vi "Display Module 2014.vi"(7 "Callling VI":refnum<vi>) -> ()   [LabVIEW 2016]
uses:
  Display Module TypeDefs/IMAQ Z Scale Bar.ctl
  <vilib>/Utility/miscctls.llb/LVPointTypeDef.ctl
  <vilib>/vision/Image Controls.llb/IMAQ Image.ctl
  <vilib>/Utility/miscctls.llb/LVRectTypeDef.ctl
  Display Module TypeDefs/Display Module Standard Action.ctl
  <vilib>/event_ctls.llb/lveventtype.ctl
  <vilib>/vision/NI_Vision_Development_Module.lvlib
panel:
  in  "Z Scale Channel 6":T1
  in  "Z Scale Channel 5":T1
  in  "Z Scale Channel 4":T1
  in  "Z Scale Channel 3":T1
  in  "Z Scale Channel 2":T1
  in  "Z Scale Channel 1":T1
  out "Messages":string
  in  "Max Left":bool
  in  "Max Right":bool
  in  "Add Display":bool
  in  "Remove Display":bool
  in  "Exit":bool
  out "Channel 6":T2(plugin-control)
  out "Channel 5":T2(plugin-control)
  out "Channel 4":T2(plugin-control)
  out "Channel 3":T2(plugin-control)
  out "Channel 2":T2(plugin-control)
  out "Channel 1":T2(plugin-control)
  # "Copyright (C) 2020 Edward S Allgeyer\n\nRedistribution and use in source and binary forms, with or without\nmodification, are permitted provided that the following conditions\nare met:\n\n1. Redistributions of source code must retain the above copyright\n   notice, this list of conditions and the following disclaimer.\n\n2. Redistributions in binary form must reproduce the above copyright\n   notice, this list of conditions and the following disclaimer in\n   the documentation and/or other materials provided with the\n   distribution.\n\n3. Neither the name of the copyright holder nor the names of its\n   contributors may be used to endorse or promote products derived\n   from this software without specific prior written permission.\n\nTHIS SOFTWARE IS PROVIDED BY THE COPYRIGHT HOLDERS AND CONTRIBUTORS\n\"AS IS\" AND ANY EXPRESS OR IMPLIED WARRANTIES, INCLUDING, BUT NOT\nLIMITED TO, THE IMPLIED WARRANTIES OF MERCHANTABILITY AND FITNESS\nFOR A PARTICULAR PURPOSE ARE DISCLAIMED. IN NO EVENT SHALL THE\nCOPYRIGHT HOLDER OR CONTRIBUTORS BE LIABLE FOR ANY DIRECT, INDIRECT,\nINCIDENTAL, SPECIAL, EXEMPLARY, OR CONSEQUENTIAL DAMAGES (INCLUDING,\nBUT NOT LIMITED TO, PROCUREMENT OF SUBSTITUTE GOODS OR SERVICES;\nLOSS OF USE, DATA, OR PROFITS; OR BUSINESS INTERRUPTION) HOWEVER\nCAUSED AND ON ANY THEORY OF LIABILITY, WHETHER IN CONTRACT, STRICT\nLIABILITY, OR TORT (INCLUDING NEGLIGENCE OR OTHERWISE) ARISING IN\nANY WAY OUT OF THE USE OF THIS SOFTWARE, EVEN IF ADVISED OF THE\nPOSSIBILITY OF SUCH DAMAGE."
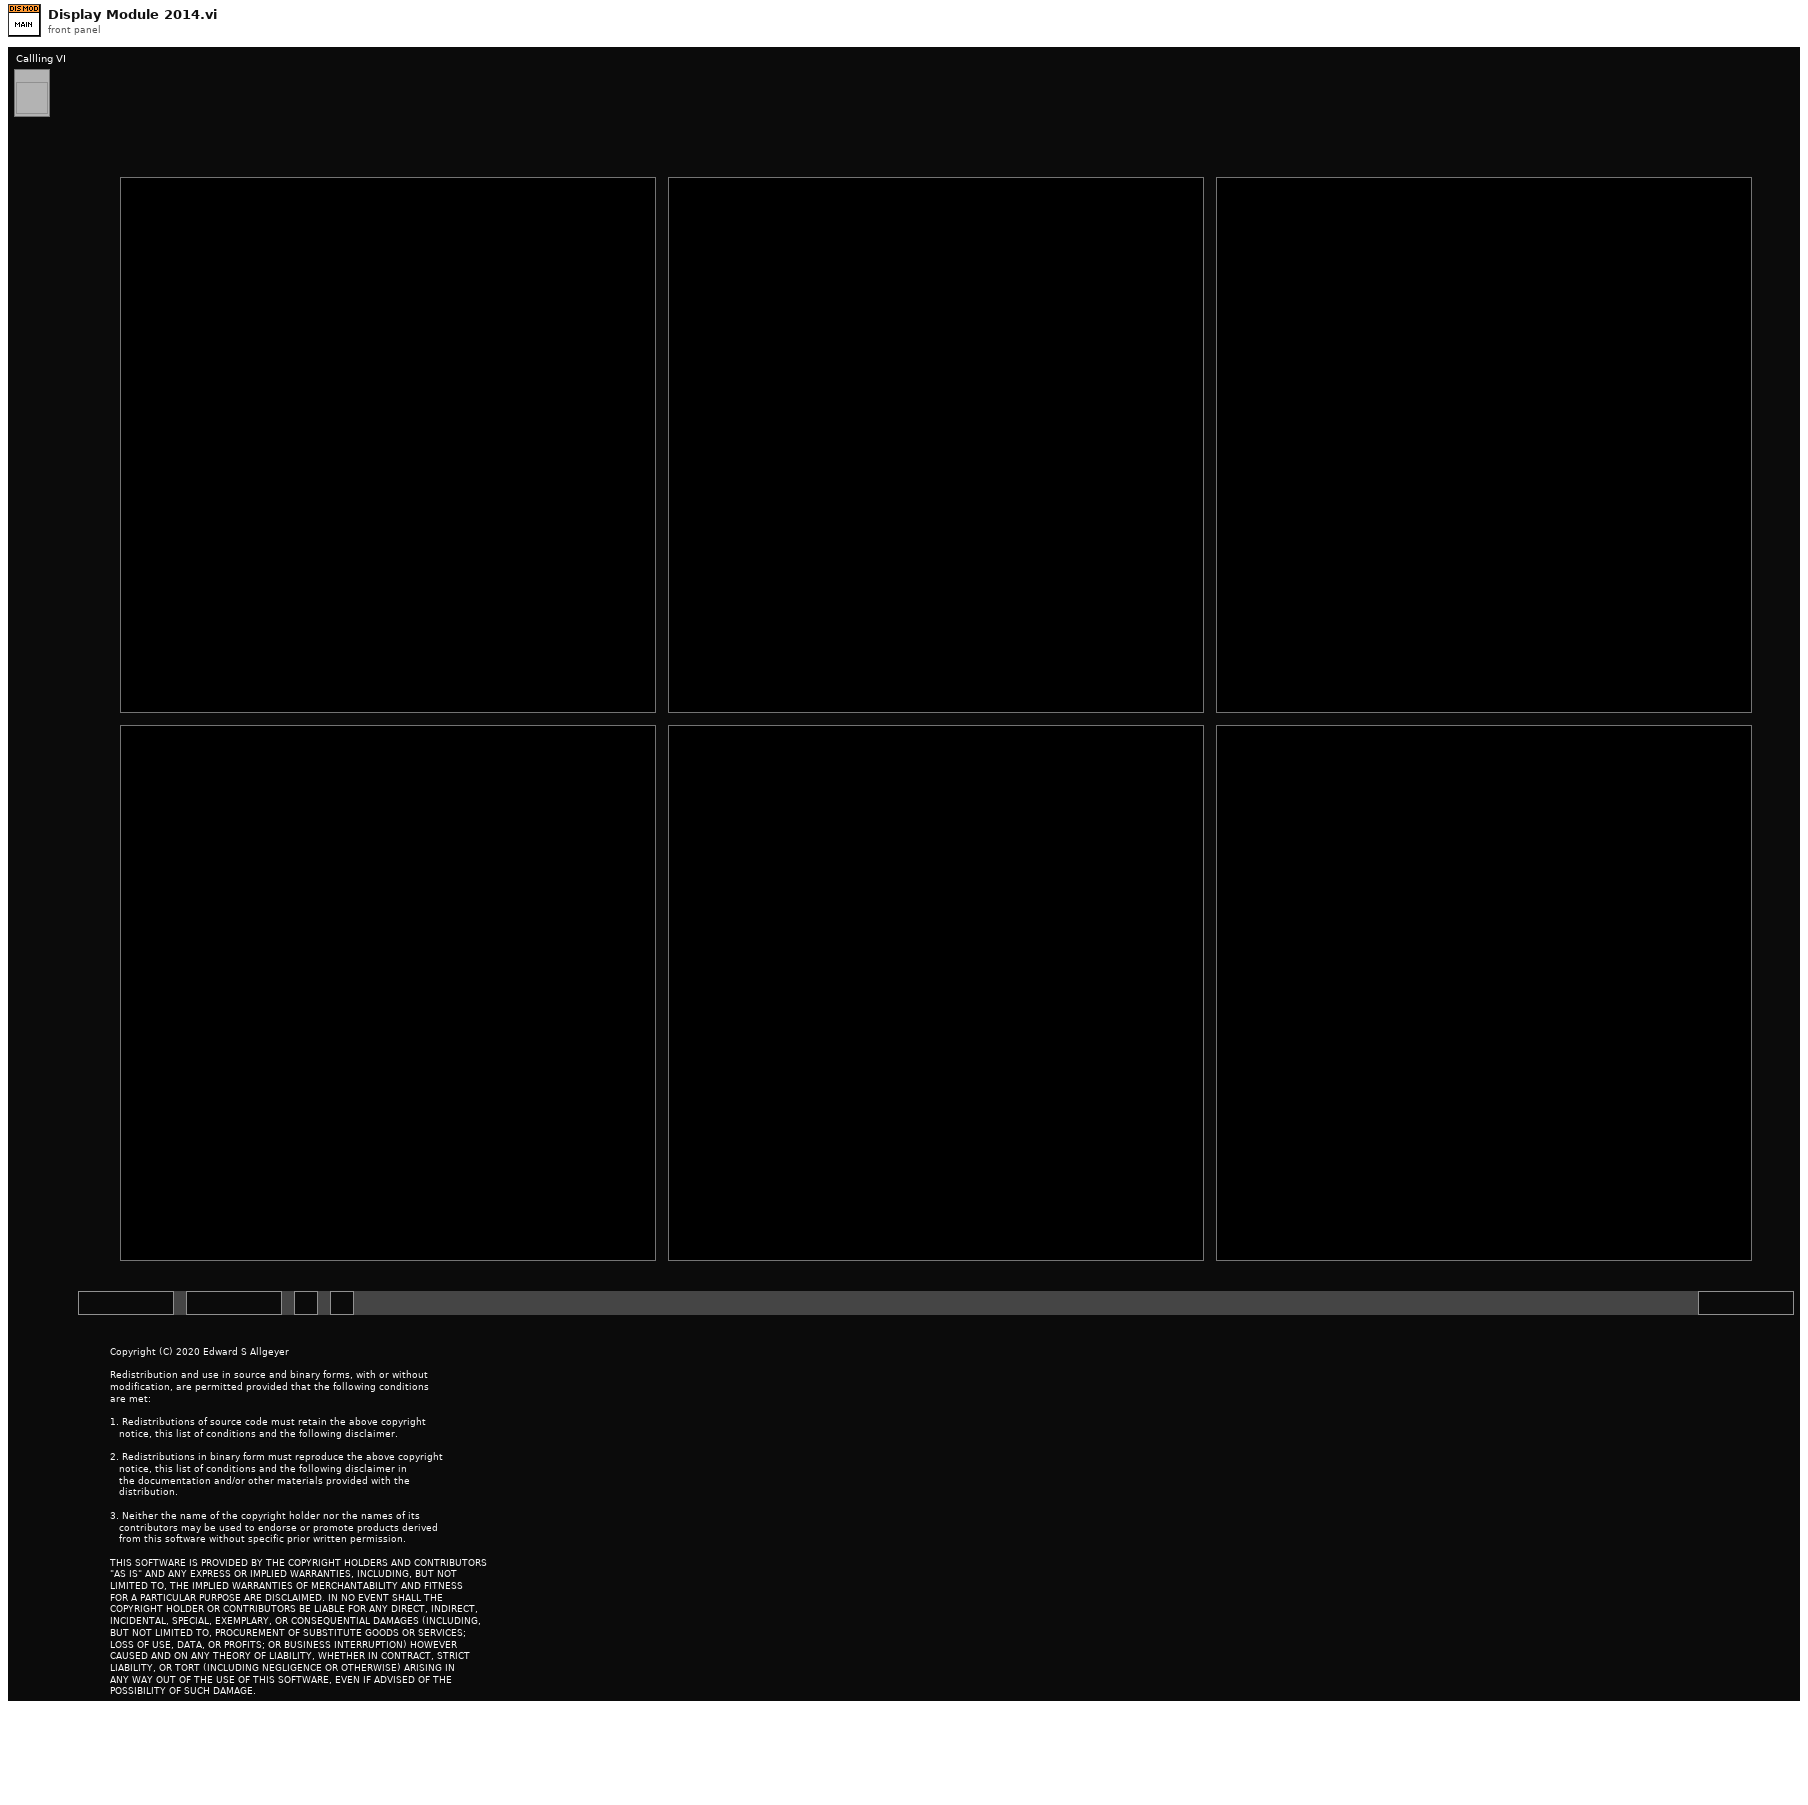
[diagram p1: front panel]
types:
  T1 = typedef "IMAQ Z Scale Bar.ctl" = cluster{"Z Scale Image":T2, "Z Scale Min":sgl, "Z Scale Max":sgl}
  T2 = typedef "IMAQ Image.ctl" = refnum<image>
  T3 = typedef "Image Type" = u32
  T4 = typedef "LVPointTypeDef.ctl" = cluster{"Horizontal":i16, "Vertical":i16}
  T5 = enum32{"Invalid", "Standard", "Closed", "Hidden", "Minimized", "Maximized"}
  T6 = enum16{"Always On", "Always Off", "Off While Running"}
  T7 = typedef "Display Module Standard Action.ctl" = enum16{"Read", "Write"}
  T8 = enum16{"Change Number", "Refresh Positions", "Get No. of Displays"}
  T9 = typedef "LVRectTypeDef.ctl" = cluster{"Left":i16, "Top":i16, "Right":i16, "Bottom":i16}
  T10 = typedef "lveventtype.ctl" = enum32{"Null", "Timeout", "Annotation Menu Selection", "Annotation Menu Selection?", "App Instance Close", "App Instance Close?", "Autoscale Range Change", "Bookmark Info Change", "Cell Edit", "Cell Edit?", "Cursor Grab", "Cursor Grab?", "Cursor Menu Selection", "Cursor Menu Selection?", "Cursor Move", "Cursor Release", "Data Change", "Direction Change", "Display State Change", "Drag Ended", "Drag Enter", "Drag Leave", "Drag Over", "Drag Source Update", "Drag Starting", "Drag Starting?", "Drop", "Exec State Change", "Key Down", "Key Down?", "Key Repeat", "Key Repeat?", "Key Up", "Listbox Double Click", "Menu Activation?", "Menu Selection (App)", "Menu Selection? (App)", "Menu Selection (User)", "Mouse Down", "Mouse Down?", "Mouse Enter", "Mouse Leave", "Mouse Move", "Mouse Up", "Mouse Wheel", "NI Security User Change (App)", "Pane Size", "Panel Close", "Panel Close?", "Panel Resize", "Plot Attribute Change", "Scale Range Change", "Shortcut Menu Activation?", "Shortcut Menu Selection (App)", "Shortcut Menu Selection? (App)", "Shortcut Menu Selection (User)", "Tree Double Click", "Tree Drag", "Tree Drag?", "Tree Drop", "Tree Drop?", "Tree Item Close", "Tree Item Close?", "Tree Item Open", "Tree Item Open?", "User Event", "Value Change"}
  T11 = cluster{"Global Rectangle":i32[], "Contours":cluster{"Contour Type":u32, "ROI Type":u32, "Points":i32[]}[]}
  T12 = typedef "LVAllMonitorsDisplayTypeDef.ctl" = cluster{"Bounds":cluster{"Left":i16, "Top":i16, "Right":i16, "Bottom":i16}, "Depth":i16}[]
  T13 = cluster{"Bounds":cluster{"Left":i16, "Top":i16, "Right":i16, "Bottom":i16}, "Depth":i16}
  T14 = cluster{"Mean Value":sgl, "Standard Variation":sgl, "Minimal Value":sgl, "Maximal Value":sgl, "Area (calibrated)":sgl, "Area (pixels)":u32, "%":sgl, "Calibration Valid":bool}
  T15 = cluster{"Contour Type":u32, "ROI Type":u32, "Points":i32[]}[]
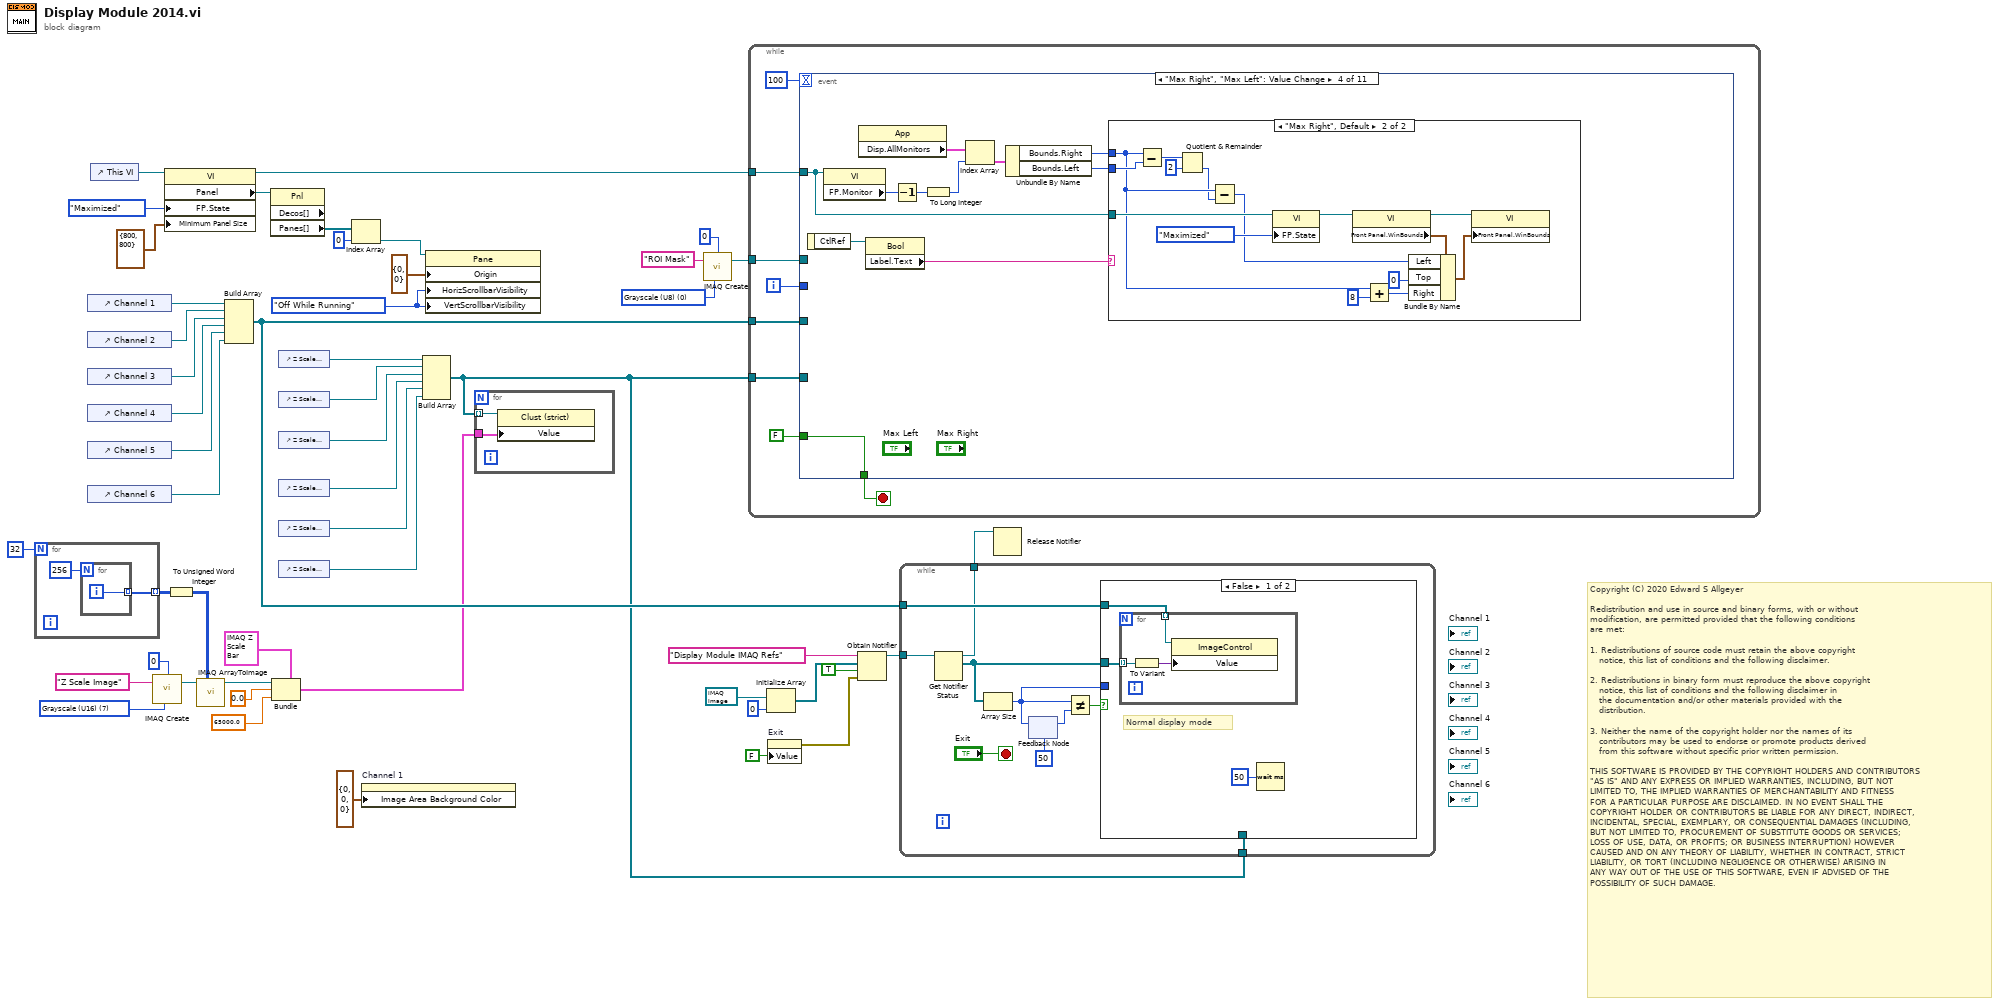
[diagram p0: block diagram]
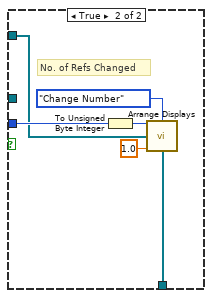
[diagram p2: hidden frame]
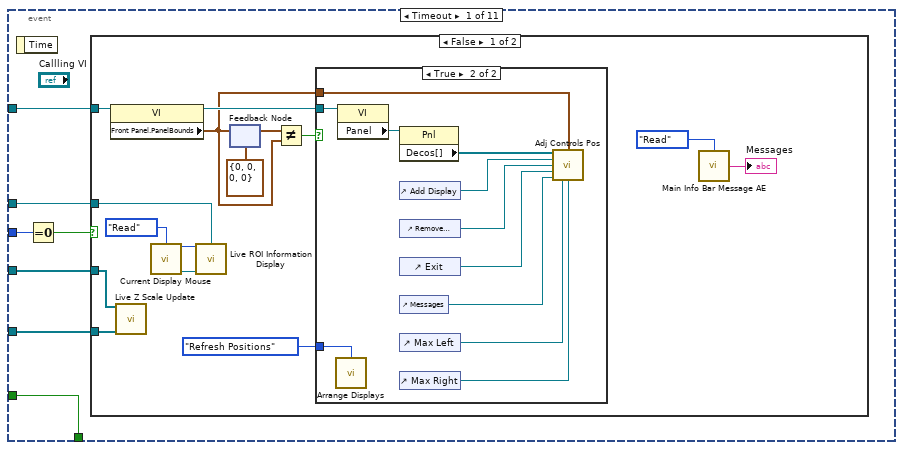
[diagram p3: hidden frame]
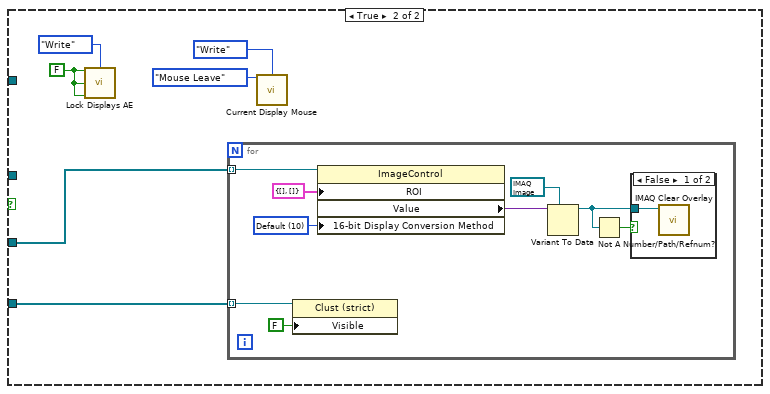
[diagram p5: hidden frame]
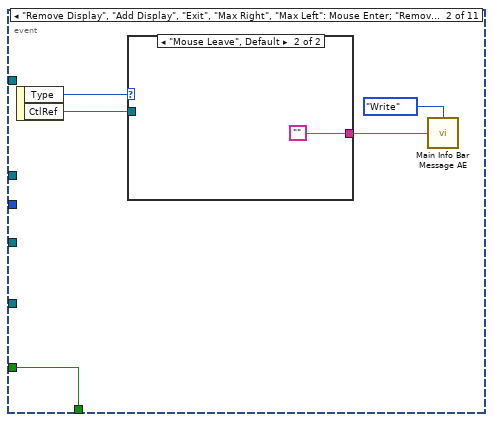
[diagram p7: hidden frame]
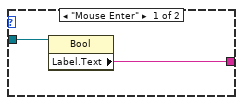
[diagram p8: hidden frame]
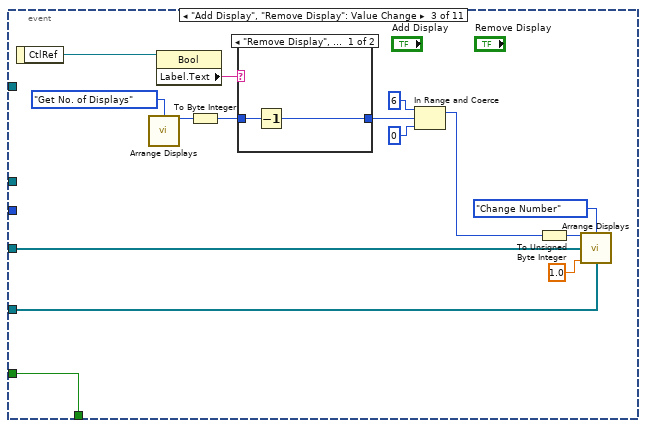
[diagram p9: hidden frame]
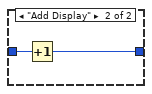
[diagram p10: hidden frame]
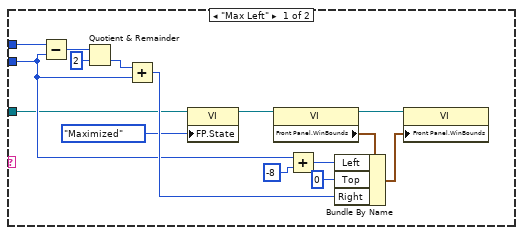
[diagram p11: hidden frame]
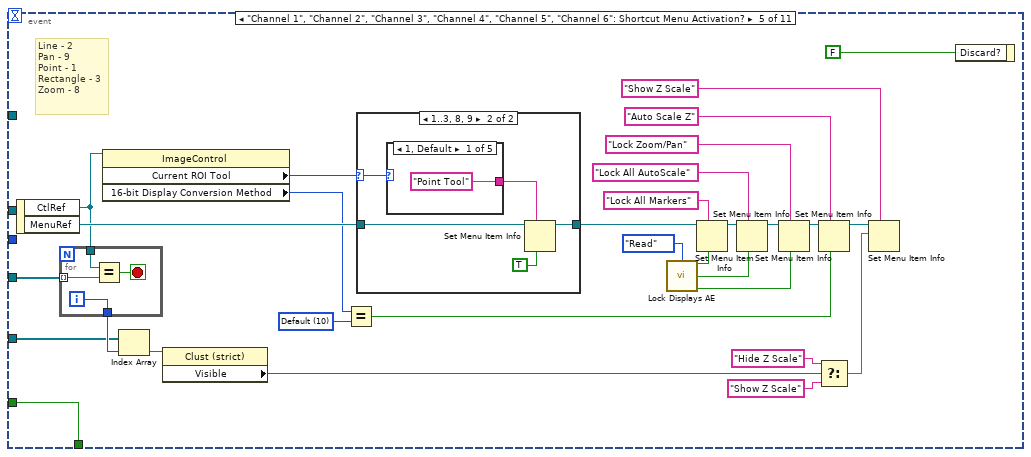
[diagram p12: hidden frame]
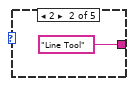
[diagram p14: hidden frame]
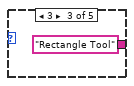
[diagram p15: hidden frame]
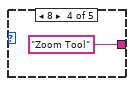
[diagram p16: hidden frame]
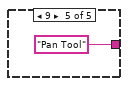
[diagram p17: hidden frame]
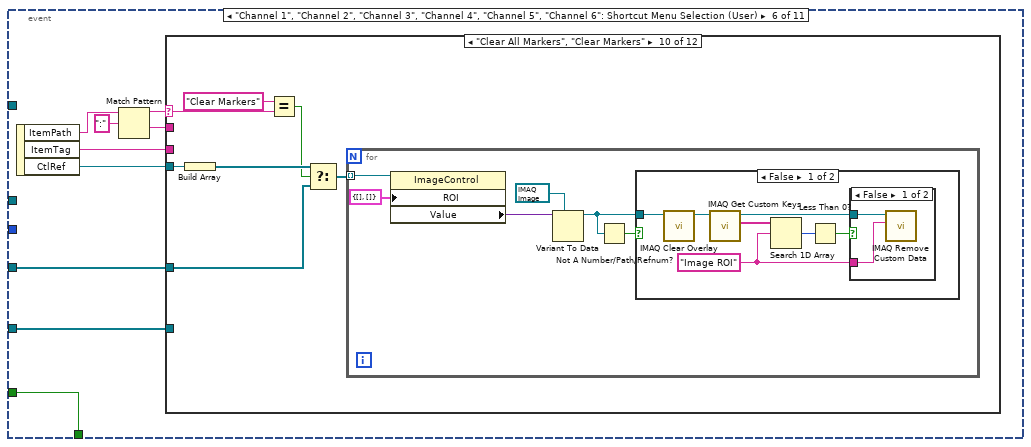
[diagram p18: hidden frame]
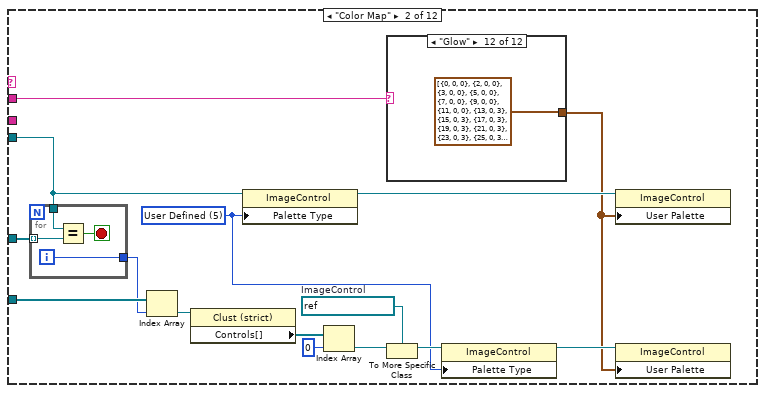
[diagram p20: hidden frame]
diagram:
  w20 = T3 7 items=["Grayscale (U8)", "Grayscale (I16)", "Grayscale (SGL)", "Complex (CSG)", "RGB (U32)", "HSL (U32)", "RGB (U64)", "Grayscale (U16)"] ("Image Type")
  w26 = T3 0 items=["Grayscale (U8)", "Grayscale (I16)", "Grayscale (SGL)", "Complex (CSG)", "RGB (U32)", "HSL (U32)", "RGB (U64)", "Grayscale (U16)"] ("Image Type")
  w41 = T6."Off While Running" ("Vertical Scrollbar Visibility")
  # "Copyright (C) 2020 Edward S Allgeyer\n\nRedistribution and use in source and binary forms, with or without\nmodification, are permitted provided that the following conditions\nare met:\n\n1. Redistributions of source code must retain the above copyright\n   notice, this list of conditions and the following disclaimer.\n\n2. Redistributions in binary form must reproduce the above copyright\n   notice, this list of conditions and the following disclaimer in\n   the documentation and/or other materials provided with the\n   distribution.\n\n3. Neither the name of the copyright holder nor the names of its\n   contributors may be used to endorse or promote products derived\n   from this software without specific prior written permission.\n\nTHIS SOFTWARE IS PROVIDED BY THE COPYRIGHT HOLDERS AND CONTRIBUTORS\n\"AS IS\" AND ANY EXPRESS OR IMPLIED WARRANTIES, INCLUDING, BUT NOT\nLIMITED TO, THE IMPLIED WARRANTIES OF MERCHANTABILITY AND FITNESS\nFOR A PARTICULAR PURPOSE ARE DISCLAIMED. IN NO EVENT SHALL THE\nCOPYRIGHT HOLDER OR CONTRIBUTORS BE LIABLE FOR ANY DIRECT, INDIRECT,\nINCIDENTAL, SPECIAL, EXEMPLARY, OR CONSEQUENTIAL DAMAGES (INCLUDING,\nBUT NOT LIMITED TO, PROCUREMENT OF SUBSTITUTE GOODS OR SERVICES;\nLOSS OF USE, DATA, OR PROFITS; OR BUSINESS INTERRUPTION) HOWEVER\nCAUSED AND ON ANY THEORY OF LIABILITY, WHETHER IN CONTRACT, STRICT\nLIABILITY, OR TORT (INCLUDING NEGLIGENCE OR OTHERWISE) ARISING IN\nANY WAY OUT OF THE USE OF THIS SOFTWARE, EVEN IF ADVISED OF THE\nPOSSIBILITY OF SUCH DAMAGE."
  n1 = for {
    N: 32 -> [_]
    tunnel: [w51] -> w18 mode=indexing
    n2 = for {
      N: 256 -> [_]
      tunnel: [w53] -> w51 mode=indexing
      i -> [w53]
    }
  }
  n3 = control-ref of="Channel 1"() -> (w50:refnum<vi>)
  n4 = control-ref of="Channel 2"() -> (w45:refnum<vi>)
  n5 = control-ref of="Channel 3"() -> (w46:refnum<vi>)
  n6 = control-ref of="Channel 4"() -> (w47:refnum<vi>)
  n7 = control-ref of="Channel 5"() -> (w48:refnum<vi>)
  n8 = control-ref of="Channel 6"() -> (w49:refnum<vi>)
  n9 = control-ref of="This VI"() -> (w40:refnum<vi>)
  n10 = call "IMAQ Create"("Border Size"=0, "Image Name"="Z Scale Image", "Image Type"=w20) -> ("New Image"=w19:T2)  [unwired: 2 in, 1 out]
  n11 = property class="VI"(reference=w40, "FP.State"=T5."Maximized" ("Front Panel Window:State"), "Minimum Panel Size"=T4 {"Horizontal"=800, "Vertical"=800} ("Front Panel Window:Minimum Size")) -> (reference out=w35:refnum<vi>, "Panel"=w36:refnum<vi>)  [unwired: 1 in, 1 out]
  n12 = To Unsigned Word Integer(number=w18) -> (unsigned 16bit integer=w17:u16[][])
  n13 = call "IMAQ ArrayToImage"("Image Pixels (U16)"=w17, "Image"=w19) -> ("Image Out"=w16:T2)  [unwired: 8 in, 1 out]
  n14 = Build Array(w50, w45, w46, w47, w48, w49) -> (w29:refnum<vi>[])
  n15 = property class="Pnl" props=["Decos[]", "Panes[]"](reference=w36) -> ("Panes[]"=w37:refnum<vi>[])  [unwired: 1 in, 3 out]
  n16 = Bundle(cluster=T1 {"Z Scale Image"="remote image 000000002503C6CC", "Z Scale Min"=0.0, "Z Scale Max"=65000.0} ("Z Scale Channel 6"), "Z Scale Image"=w16, "Z Scale Min"=sgl 0.0, "Z Scale Max"=sgl 65000.0) -> (w7:T1)
  n17 = control-ref of="Z Scale Channel 1"() -> (w13:refnum<vi>)
  n18 = control-ref of="Z Scale Channel 2"() -> (w8:refnum<vi>)
  n19 = control-ref of="Z Scale Channel 3"() -> (w9:refnum<vi>)
  n20 = control-ref of="Z Scale Channel 4"() -> (w10:refnum<vi>)
  n21 = control-ref of="Z Scale Channel 5"() -> (w11:refnum<vi>)
  n22 = control-ref of="Z Scale Channel 6"() -> (w12:refnum<vi>)
  n23 = Index Array(array=w37, index=0) -> (element=w43:refnum<vi>)
  n24 = property on="Channel 1" class="ImageControl"("Image Area Background Color"=cluster{"Red":u8, "Green":u8, "Blue":u8} {"Red"=0, "Green"=0, "Blue"=0} ("Image Area:Background:Background Color")) -> ()  [unwired: 2 in, 2 out]
  n25 = Build Array(w13, w8, w9, w10, w11, w12) -> (w5:refnum<vi>[])
  n26 = property class="Pane"(reference=w43, "Origin"=T4 {"Horizontal"=0, "Vertical"=0}, "HorizScrollbarVisibility"=w41, "VertScrollbarVisibility"=w41) -> ()  [unwired: 1 in, 2 out]
  n27 = for {
    tunnel: w5 -> [w55] mode=indexing
    tunnel: w7 -> [w54]
    n28 = property class="Clust (strict)"(reference=w55, "Value"=w54) -> ()  [unwired: 1 in, 2 out]
  }
  n29 = call "IMAQ Create"("Border Size"=0, "Image Name"="ROI Mask", "Image Type"=w26) -> ("New Image"=w24:T2)  [unwired: 2 in, 1 out]
  n30 = while {
    tunnel: w29 -> [w62]
    tunnel: w35 -> [w58]
    tunnel: w24 -> [w57]
    tunnel: w5 -> [w56]
    i -> [w63]
    stop <- w61 stop-if-true
    n31 = event shown="[3] \"Max Right\", \"Max Left\": Value Change" {
      selector: _ -> [_ _ _ _ _ _ _ _ _ _ _]
      dyn-events: _ -> [_ _ _ _ _ _ _ _ _ _ _]
      timeout: 100 -> [_ _ _ _ _ _ _ _ _ _ _]
      tunnel: w63 -> [w70 _ _ _ _ _ _ _ _ _ _]
      tunnel: w62 -> [w68 _ w122 _ w185 w228 w397 _ w433 w441 w458]
      tunnel: [w67 w117 w135 w150 w209 w234 w402 w424 w435 w447 w459] -> w61
      tunnel: FALSE -> [w67 w117 w135 w150 w209 w234 w402 w424 w435 w447 _]
      tunnel: w58 -> [w66 _ _ w141 _ _ _ _ _ _ _]
      tunnel: w57 -> [w65 _ _ _ _ _ _ _ _ _ w457]
      tunnel: w56 -> [w64 _ w123 _ w186 w227 _ _ w434 _ _]
      event Timeout {
        n32 = event-data() -> ()  [unwired: 1 in, 1 out]
        n33 = Equal To 0?(x=w70) -> (x = 0?=w69:bool)
        n34 = case shown="False" w69 {
          tunnel: w68 -> [w72 w100]
          tunnel: w66 -> [w85 _]
          tunnel: w65 -> [w78 _]
          tunnel: w64 -> [w71 w99]
          frame False {
            n35 = property class="VI"(reference=w85) -> (reference out=w81:refnum<vi>, "Front Panel.PanelBounds"=w80:T9)  [unwired: 1 in, 1 out]
            n36 = call "Live Z Scale Update.vi"("IMAQ Display Refs"=w72, "Z Scale Refs"=w71) -> ()  [unwired: 14 in]
            n37 = call "Current Display Mouse.vi"("Action"=Display_Module_Standard_Action."Read") -> ("Event Type Out"=w76:T10, "IMAQ Image Display Ref Out"=w75:refnum<vi>)  [unwired: 13 in]
            n38 = call "Live ROI Information Display.vi"("Event Type"=w76, "ROI Mask REF"=w78, "IMAQ Image Display Ref"=w75) -> ()  [unwired: 13 in]
            n39 = feedback-in #1(w80) -> ()
            n40 = feedback #1(T9 {"Left"=0, "Top"=0, "Right"=0, "Bottom"=0} ("Front Panel.PanelBounds")) -> (w84:T9)
            n41 = Not Equal?(x=w84, y=w80) -> (x != y?=w82:bool)
            n42 = case shown="True" w82 {
              tunnel: w81 -> [_ w90]
              tunnel: w80 -> [_ w89]
              tunnel: T8."Refresh Positions" ("Action") -> [_ w86]
              frame False {
              }
              frame True {
                n43 = call "Arrange Displays.vi"("Action"=w86) -> ()  [unwired: 13 in, 2 out]
                n44 = property class="VI"(reference=w90) -> ("Panel"=w96:refnum<vi>)  [unwired: 1 in, 2 out]
                n45 = property class="Pnl"(reference=w96) -> ("Decos[]"=w95:refnum<vi>[])  [unwired: 1 in, 2 out]
                n46 = control-ref of="Add Display"() -> (w91:refnum<vi>)
                n47 = control-ref of="Remove Display"() -> (w94:refnum<vi>)
                n48 = control-ref of="Exit"() -> (w93:refnum<vi>)
                n49 = control-ref of="Messages"() -> (w92:refnum<vi>)
                n50 = control-ref of="Max Left"() -> (w88:refnum<vi>)
                n51 = control-ref of="Max Right"() -> (w87:refnum<vi>)
                n52 = call "Adj Controls Pos.vi"("Decoration Ref Array"=w95, "Panel Bounds"=w89, "Add Display Ref (Bool)"=w91, "Remove Display Ref (Bool)"=w94, "Exit (Bool)"=w93, "Message (String)"=w92, "Max Left (Bool)"=w88, "Max Right (Bool)"=w87) -> ()  [unwired: 8 in]
              }
            }
            n53 = call "Main Info Bar Message AE.vi"("Action"=Display_Module_Standard_Action."Read") -> ("Message Out"=→"Messages":string)  [unwired: 14 in]
          }
          frame True {
            w102 = FALSE ("Lock All Markers")
            n54 = call "Lock Displays AE.vi"("Lock All Markers"=w102, "Action"=Display_Module_Standard_Action."Write", "Lock All AutoScale"=w102, "Lock Pan/Zoom"=w102) -> ()  [unwired: 9 in, 3 out]
            n55 = for {
              tunnel: w100 -> [w106] mode=indexing
              tunnel: w99 -> [w105] mode=indexing
              w103 = u32 10 items=["Default"=10, "Most Significant Bits"=11, "Full Dynamic"=12, "Downshift"=13, "Given Range"=14, "90% Dynamic"=15, "Given Percent Range"=16] ("16-bit Display Mapping:Conversion Method")
              n56 = property class="Clust (strict)"(reference=w105, "Visible"=FALSE) -> ()  [unwired: 1 in, 2 out]
              n57 = property class="ImageControl"(reference=w106, "ROI"=T11 {"Global Rectangle"=[], "Contours"=[]}, "16-bit Display Conversion Method"=w103) -> ("Value"=w107:variant)  [unwired: 1 in, 2 out]
              n58 = Variant To Data(type=T2 refnum ("New Image"), Variant=w107) -> (data=w110:T2)  [unwired: 1 in, 1 out]
              n59 = Not A Number/Path/Refnum?(number/path/refnum=w110) -> (NaN/Path/Refnum?=w109:bool)
              n60 = case shown="False" w109 {
                tunnel: w110 -> [w112 _]
                frame False {
                  n61 = call "IMAQ Clear Overlay"("Image"=w112) -> ()  [unwired: 9 in, 2 out]
                }
                frame True {
                }
              }
            }
            n62 = call "Current Display Mouse.vi"("Event Type"=lveventtype."Mouse Leave", "Action"=Display_Module_Standard_Action."Write") -> ()  [unwired: 12 in, 2 out]
          }
        }
      }
      event "Remove Display", "Add Display", "Exit", "Max Right", "Max Left": Mouse Enter; "Remove Display", "Add Display", "Exit", "Max Right", "Max Left": Mouse Leave {
        n63 = event-data() -> ("Type"=w116:T10, "CtlRef"=w115:refnum<vi>)  [unwired: 1 in]
        n64 = case shown="\"Mouse Leave\", Default" w116 {
          tunnel: w115 -> [w119 _]
          tunnel: [w118 ""] -> w113
          frame "Mouse Enter" {
            n65 = property class="Bool"(reference=w119) -> ("Label.Text"=w118:string)  [unwired: 1 in, 2 out]
          }
          frame "Mouse Leave", Default {
          }
        }
        n66 = call "Main Info Bar Message AE.vi"("Action"=Display_Module_Standard_Action."Write", "Message"=w113) -> ()  [unwired: 13 in, 1 out]
      }
      event "Add Display", "Remove Display": Value Change {
        n67 = event-data() -> ("CtlRef"=w134:refnum<vi>)  [unwired: 1 in]
        n68 = call "Arrange Displays.vi"("Action"=T8."Get No. of Displays") -> ("Number of Displays Out"=w125:u8)  [unwired: 13 in, 1 out]
        n69 = property class="Bool"(reference=w134) -> ("Label.Text"=w133:string)  [unwired: 1 in, 2 out]
        n70 = To Byte Integer(number=w125) -> (8bit integer=w124:i8)
        n71 = case shown="\"Remove Display\", Default" w133 {
          tunnel: w124 -> [w137 w139]
          tunnel: [w136 w138] -> w130
          frame "Remove Display", Default {
            n72 = Decrement(x=w137) -> (x-1=w136:i8)
          }
          frame "Add Display" {
            n73 = Increment(x=w139) -> (x+1=w138:i8)
          }
        }
        n74 = In Range and Coerce(upper limit=i8 6, x=w130, lower limit=i8 0) -> (coerced(x)=w129:i8)  [unwired: 1 out]
        n75 = To Unsigned Byte Integer(number=w129) -> (unsigned 8bit integer=w128:u8)
        n76 = call "Arrange Displays.vi"("Number of Displays"=w128, "Action"=T8."Change Number", "IMAQ Display Refs"=w122, "Aspect Ratio (Width/Height)"=1.0, "Z Scale Refs"=w123) -> ()  [unwired: 9 in, 2 out]
      }
      event "Max Right", "Max Left": Value Change {
        n77 = event-data() -> ("CtlRef"=w149:refnum<vi>)  [unwired: 1 in]
        n78 = property class="VI"(reference=w141) -> ("FP.Monitor"=w148:u16)  [unwired: 1 in, 2 out]
        n79 = property class="App"() -> ("Disp.AllMonitors"=w147:T12)  [unwired: 2 in, 2 out]
        n80 = property class="Bool"(reference=w149) -> ("Label.Text"=w140:string)  [unwired: 1 in, 2 out]
        n81 = Decrement(x=w148) -> (x-1=w146:u16)
        n82 = To Long Integer(number=w146) -> (32bit integer=w145:i32)
        n83 = Index Array(array=w147, index=w145) -> (element=w144:T13)
        n84 = Unbundle By Name(w144) -> ("Bounds.Right"=w143:i16, "Bounds.Left"=w142:i16)
        n85 = case shown="\"Max Right\", Default" w140 {
          tunnel: w143 -> [w165 w168]
          tunnel: w142 -> [w153 w172]
          tunnel: w141 -> [w151 w171]
          frame "Max Left" {
            n86 = Subtract(x=w165, y=w153) -> (x-y=w160:i16)
            n87 = Quotient & Remainder(x=w160, y=i16 2) -> (floor(x/y)=w158:i16)  [unwired: 1 out]
            n88 = Add(x=w158, y=w153) -> (x+y=w157:i16)
            n89 = property class="VI"(reference=w151, "FP.State"=T5."Maximized" ("Front Panel Window:State")) -> (reference out=w155:refnum<vi>)  [unwired: 1 in, 1 out]
            n90 = property class="VI"(reference=w155) -> (reference out=w164:refnum<vi>, "Front Panel.WinBounds"=w162:T9)  [unwired: 1 in, 1 out]
            n91 = Add(x=w153, y=i16 -8 ("Left")) -> (x+y=w152:i16)
            n92 = Bundle By Name(cluster=w162, "Left"=w152, "Top"=i16 0, "Right"=w157) -> (w163:T9)
            n93 = property class="VI"(reference=w164, "Front Panel.WinBounds"=w163) -> ()  [unwired: 1 in, 2 out]
          }
          frame "Max Right", Default {
            n94 = Subtract(x=w168, y=w172) -> (x-y=w177:i16)
            n95 = Quotient & Remainder(x=w177, y=i16 2) -> (floor(x/y)=w167:i16)  [unwired: 1 out]
            n96 = Subtract(x=w168, y=w167) -> (x-y=w166:i16)
            n97 = property class="VI"(reference=w171, "FP.State"=T5."Maximized" ("Front Panel Window:State")) -> (reference out=w174:refnum<vi>)  [unwired: 1 in, 1 out]
            n98 = property class="VI"(reference=w174) -> (reference out=w180:refnum<vi>, "Front Panel.WinBounds"=w178:T9)  [unwired: 1 in, 1 out]
            n99 = Add(x=w168, y=i16 8 ("Left")) -> (x+y=w169:i16)
            n100 = Bundle By Name(cluster=w178, "Left"=w166, "Top"=i16 0, "Right"=w169) -> (w179:T9)
            n101 = property class="VI"(reference=w180, "Front Panel.WinBounds"=w179) -> ()  [unwired: 1 in, 2 out]
          }
        }
      }
      event "Channel 1", "Channel 2", "Channel 3", "Channel 4", "Channel 5", "Channel 6": Shortcut Menu Activation? {
        w192 = u32 10 items=["Default"=10, "Most Significant Bits"=11, "Full Dynamic"=12, "Downshift"=13, "Given Range"=14, "90% Dynamic"=15, "Given Percent Range"=16] ("16-bit Display Mapping:Conversion Method")
        # "Line - 2\nPan - 9\nPoint - 1\nRectangle - 3\nZoom - 8"
        n102 = event-data() -> ("CtlRef"=w187:refnum<vi>, "MenuRef"=w207:refnum<k9>)  [unwired: 1 in]
        n103 = for {
          tunnel: w185 -> [w214] mode=indexing
          tunnel: w187 -> [w212]
          tunnel: [w211] -> w189
          i -> [w211]
          stop <- w213 stop-if-true
          n104 = Equal?(x=w212, y=w214) -> (x = y?=w213:bool)
        }
        n105 = property class="ImageControl"(reference=w187) -> ("Current ROI Tool"=w208:u32, "16-bit Display Conversion Method"=w194:u32)  [unwired: 1 in, 2 out]
        n106 = Index Array(array=w186, index=w189) -> (element=w188:refnum<vi>)
        n107 = property class="Clust (strict)"(reference=w188) -> ("Visible"=w181:bool)  [unwired: 1 in, 2 out]
        n108 = Equal?(x=w194, y=w192) -> (x = y?=w193:bool)
        n109 = case shown="1..3, 8, 9" w208 {
          selector: w208 -> [_ w220]
          tunnel: w207 -> [w215 w218]
          tunnel: [w215 w216] -> w206
          frame Default {
          }
          frame 1..3, 8, 9 {
            n110 = case shown="1, Default" w220 {
              tunnel: ["Point Tool" ("item tag") "Line Tool" ("item tag") "Rectangle Tool" ("item tag") "Zoom Tool" ("item tag") "Pan Tool" ("item tag")] -> w217
              frame 1, Default {
              }
              frame 2 {
              }
              frame 3 {
              }
              frame 8 {
              }
              frame 9 {
              }
            }
            n111 = Set Menu Item Info(6:TRUE ("checked"), 7:w217, 11:w218) -> (3:w216:refnum<k9>)  [unwired: 4 in, 1 out]
          }
        }
        n112 = call "Lock Displays AE.vi"("Action"=Display_Module_Standard_Action."Read") -> ("Lock All Markers Out"=w199:bool, "Lock All AutoScale Out"=w198:bool, "Lock Pan/Zoom Out"=w197:bool)  [unwired: 12 in]
        n113 = Set Menu Item Info(6:w199, 7:"Lock All Markers" ("item tag"), 11:w206) -> (3:w205:refnum<k9>)  [unwired: 4 in, 1 out]
        n114 = Set Menu Item Info(6:w198, 7:"Lock All AutoScale" ("item tag"), 11:w205) -> (3:w204:refnum<k9>)  [unwired: 4 in, 1 out]
        n115 = Set Menu Item Info(6:w197, 7:"Lock Zoom/Pan" ("item tag"), 11:w204) -> (3:w196:refnum<k9>)  [unwired: 4 in, 1 out]
        n116 = Set Menu Item Info(6:w193, 7:"Auto Scale Z" ("item tag"), 11:w196) -> (3:w191:refnum<k9>)  [unwired: 4 in, 1 out]
        n117 = Select(t="Hide Z Scale" ("item tag"), s=w181, f="Show Z Scale" ("item tag")) -> (s? t:f=w182:string)
        n118 = Set Menu Item Info(7:"Show Z Scale" ("item tag"), 10:w182, 11:w191) -> ()  [unwired: 4 in, 2 out]
        n119 = event-data("Discard?"=FALSE) -> ()  [unwired: 1 in, 1 out]
      }
      event "Channel 1", "Channel 2", "Channel 3", "Channel 4", "Channel 5", "Channel 6": Shortcut Menu Selection (User) {
        n120 = event-data() -> ("ItemPath"=w232:string, "ItemTag"=w233:string, "CtlRef"=w229:refnum<vi>)  [unwired: 1 in]
        n121 = Match Pattern(string=w232, regular expression=":") -> (before substring=w230:string, after substring=w226:string)  [unwired: 1 in, 2 out]
        n122 = case shown="\"Clear All Markers\", \"Clear Markers\"" w230 {
          selector: w230 -> [_ _ w267 _ _ _ _ _ _ w363 _ _]
          tunnel: w229 -> [_ w247 w273 w298 _ w320 _ w334 w344 w361 w385 _]
          tunnel: w233 -> [_ _ _ _ _ _ _ _ _ _ _ _]
          tunnel: w228 -> [_ w248 _ w301 w312 w322 _ w333 w345 w359 w381 _]
          tunnel: w227 -> [_ w246 _ w300 _ w321 _ _ _ _ _ _]
          tunnel: w226 -> [_ w235 _ _ _ _ _ _ _ _ _ _]
          frame Default {
          }
          frame "Color Map" {
            w241 = refnum<vi> refnum  # ImageControl
            w237 = u32 5 items=["Grayscale", "Binary", "Gradient", "Rainbow", "Temperature", "User Defined", "Binary 16 Bit", "Gradient 16 Bit", "Rainbow 16 Bit", "Temperature 16 Bit", "User Defined 16 Bit"] ("Palette:Palette Type")
            n123 = for {
              tunnel: w248 -> [w264] mode=indexing
              tunnel: [w265] -> w245
              tunnel: w247 -> [w263]
              i -> [w265]
              stop <- w262 stop-if-true
              n124 = Equal?(x=w263, y=w264) -> (x = y?=w262:bool)
            }
            n125 = Index Array(array=w246, index=w245) -> (element=w244:refnum<vi>)
            n126 = property class="Clust (strict)"(reference=w244) -> ("Controls[]"=w243:refnum<vi>[])  [unwired: 1 in, 2 out]
            n127 = property class="ImageControl"(reference=w247, "Palette Type"=w237) -> (reference out=w249:refnum<vi>)  [unwired: 1 in, 1 out]
            n128 = Index Array(array=w243, index=0) -> (element=w240:refnum<vi>)
            n129 = case shown="\"Glow\"" w235 {
              tunnel: [cluster{u8, u8, u8}[] [{0, 0, 0}, {1, 1, 1}, {2, 2, 2}, {3, 3, 3}, {4, 4, 4}, {5, 5, 5}, {6, 6, 6}, {7, 7, 7}, {8, 8, 8}, {9, 9, 9}, {10, 10, 10}, {11, 11, 11}, {12, 12, 12}, {13, 13, 13}, {14, 14, 14}, {15, 15, 15}, {16, 16, 16}, {17, 17, 17}, {18, 18, 18}, {19, 19, 19}, {20, 20, 20}, {21, 21, 21}, {22, 22, 22}, {23, 23, 23}, {24, 24, 24}, {25, 25, 25}, {26, 26, 26}, {27, 27, 27}, {28, 28, 28}, {29, 29, 29}, {30, 30, 30}, {31, 31, 31}, {32, 32, 32}, {33, 33, 33}, {34, 34, 34}, {35, 35, 35}, {36, 36, 36}, {37, 37, 37}, {38, 38, 38}, {39, 39, 39}, {40, 40, 40}, {41, 41, 41}, {42, 42, 42}, {43, 43, 43}, {44, 44, 44}, {45, 45, 45}, {46, 46, 46}, {47, 47, 47}, {48, 48, 48}, {49, 49, 49}, {50, 50, 50}, {51, 51, 51}, {52, 52, 52}, {53, 53, 53}, {54, 54, 54}, {55, 55, 55}, {56, 56, 56}, {57, 57, 57}, {58, 58, 58}, {59, 59, 59}, {60, 60, 60}, {61, 61, 61}, {62, 62, 62}, {63, 63, 63}, {64, 64, 64}, {65, 65, 65}, {66, 66, 66}, {67, 67, 67}, {68, 68, 68}, {69, 69, 69}, {70, 70, 70}, {71, 71, 71}, {72, 72, 72}, {73, 73, 73}, {74, 74, 74}, {75, 75, 75}, {76, 76, 76}, {77, 77, 77}, {78, 78, 78}, {79, 79, 79}, {80, 80, 80}, {81, 81, 81}, {82, 82, 82}, {83, 83, 83}, {84, 84, 84}, {85, 85, 85}, {86, 86, 86}, {87, 87, 87}, {88, 88, 88}, {89, 89, 89}, {90, 90, 90}, {91, 91, 91}, {92, 92, 92}, {93, 93, 93}, {94, 94, 94}, {95, 95, 95}, {96, 96, 96}, {97, 97, 97}, {98, 98, 98}, {99, 99, 99}, {100, 100, 100}, {101, 101, 101}, {102, 102, 102}, {103, 103, 103}, {104, 104, 104}, {105, 105, 105}, {106, 106, 106}, {107, 107, 107}, {108, 108, 108}, {109, 109, 109}, {110, 110, 110}, {111, 111, 111}, {112, 112, 112}, {113, 113, 113}, {114, 114, 114}, {115, 115, 115}, {116, 116, 116}, {117, 117, 117}, {118, 118, 118}, {119, 119, 119}, {120, 120, 120}, {121, 121, 121}, {122, 122, 122}, {123, 123, 123}, {124, 124, 124}, {125, 125, 125}, {126, 126, 126}, {127, 127, 127}, {128, 128, 128}, {129, 129, 129}, {130, 130, 130}, {131, 131, 131}, {132, 132, 132}, {133, 133, 133}, {134, 134, 134}, {135, 135, 135}, {136, 136, 136}, {137, 137, 137}, {138, 138, 138}, {139, 139, 139}, {140, 140, 140}, {141, 141, 141}, {142, 142, 142}, {143, 143, 143}, {144, 144, 144}, {145, 145, 145}, {146, 146, 146}, {147, 147, 147}, {148, 148, 148}, {149, 149, 149}, {150, 150, 150}, {151, 151, 151}, {152, 152, 152}, {153, 153, 153}, {154, 154, 154}, {155, 155, 155}, {156, 156, 156}, {157, 157, 157}, {158, 158, 158}, {159, 159, 159}, {160, 160, 160}, {161, 161, 161}, {162, 162, 162}, {163, 163, 163}, {164, 164, 164}, {165, 165, 165}, {166, 166, 166}, {167, 167, 167}, {168, 168, 168}, {169, 169, 169}, {170, 170, 170}, {171, 171, 171}, {172, 172, 172}, {173, 173, 173}, {174, 174, 174}, {175, 175, 175}, {176, 176, 176}, {177, 177, 177}, {178, 178, 178}, {179, 179, 179}, {180, 180, 180}, {181, 181, 181}, {182, 182, 182}, {183, 183, 183}, {184, 184, 184}, {185, 185, 185}, {186, 186, 186}, {187, 187, 187}, {188, 188, 188}, {189, 189, 189}, {190, 190, 190}, {191, 191, 191}, {192, 192, 192}, {193, 193, 193}, {194, 194, 194}, {195, 195, 195}, {196, 196, 196}, {197, 197, 197}, {198, 198, 198}, {199, 199, 199}, {200, 200, 200}, {201, 201, 201}, {202, 202, 202}, {203, 203, 203}, {204, 204, 204}, {205, 205, 205}, {206, 206, 206}, {207, 207, 207}, {208, 208, 208}, {209, 209, 209}, {210, 210, 210}, {211, 211, 211}, {212, 212, 212}, {213, 213, 213}, {214, 214, 214}, {215, 215, 215}, {216, 216, 216}, {217, 217, 217}, {218, 218, 218}, {219, 219, 219}, {220, 220, 220}, {221, 221, 221}, {222, 222, 222}, {223, 223, 223}, {224, 224, 224}, {225, 225, 225}, {226, 226, 226}, {227, 227, 227}, {228, 228, 228}, {229, 229, 229}, {230, 230, 230}, {231, 231, 231}, {232, 232, 232}, {233, 233, 233}, {234, 234, 234}, {235, 235, 235}, {236, 236, 236}, {237, 237, 237}, {238, 238, 238}, {239, 239, 239}, {240, 240, 240}, {241, 241, 241}, {242, 242, 242}, {243, 243, 243}, {244, 244, 244}, {245, 245, 245}, {246, 246, 246}, {247, 247, 247}, {248, 248, 248}, {249, 249, 249}, {250, 250, 250}, {251, 251, 251}, {252, 252, 252}, {253, 253, 253}, {254, 254, 254}, {255, 255, 255}] ("Array") cluster{u8, u8, u8}[] [{0, 0, 0}, {1, 0, 0}, {2, 0, 0}, {3, 0, 0}, {4, 0, 0}, {5, 0, 0}, {6, 0, 0}, {7, 0, 0}, {8, 0, 0}, {9, 0, 0}, {10, 0, 0}, {11, 0, 0}, {12, 0, 0}, {13, 0, 0}, {14, 0, 0}, {15, 0, 0}, {16, 0, 0}, {17, 0, 0}, {18, 0, 0}, {19, 0, 0}, {20, 0, 0}, {21, 0, 0}, {22, 0, 0}, {23, 0, 0}, {24, 0, 0}, {25, 0, 0}, {26, 0, 0}, {27, 0, 0}, {28, 0, 0}, {29, 0, 0}, {30, 0, 0}, {31, 0, 0}, {32, 0, 0}, {33, 0, 0}, {34, 0, 0}, {35, 0, 0}, {36, 0, 0}, {37, 0, 0}, {38, 0, 0}, {39, 0, 0}, {40, 0, 0}, {41, 0, 0}, {42, 0, 0}, {43, 0, 0}, {44, 0, 0}, {45, 0, 0}, {46, 0, 0}, {47, 0, 0}, {48, 0, 0}, {49, 0, 0}, {50, 0, 0}, {51, 0, 0}, {52, 0, 0}, {53, 0, 0}, {54, 0, 0}, {55, 0, 0}, {56, 0, 0}, {57, 0, 0}, {58, 0, 0}, {59, 0, 0}, {60, 0, 0}, {61, 0, 0}, {62, 0, 0}, {63, 0, 0}, {64, 0, 0}, {65, 0, 0}, {66, 0, 0}, {67, 0, 0}, {68, 0, 0}, {69, 0, 0}, {70, 0, 0}, {71, 0, 0}, {72, 0, 0}, {73, 0, 0}, {74, 0, 0}, {75, 0, 0}, {76, 0, 0}, {77, 0, 0}, {78, 0, 0}, {79, 0, 0}, {80, 0, 0}, {81, 0, 0}, {82, 0, 0}, {83, 0, 0}, {84, 0, 0}, {85, 0, 0}, {86, 0, 0}, {87, 0, 0}, {88, 0, 0}, {89, 0, 0}, {90, 0, 0}, {91, 0, 0}, {92, 0, 0}, {93, 0, 0}, {94, 0, 0}, {95, 0, 0}, {96, 0, 0}, {97, 0, 0}, {98, 0, 0}, {99, 0, 0}, {100, 0, 0}, {101, 0, 0}, {102, 0, 0}, {103, 0, 0}, {104, 0, 0}, {105, 0, 0}, {106, 0, 0}, {107, 0, 0}, {108, 0, 0}, {109, 0, 0}, {110, 0, 0}, {111, 0, 0}, {112, 0, 0}, {113, 0, 0}, {114, 0, 0}, {115, 0, 0}, {116, 0, 0}, {117, 0, 0}, {118, 0, 0}, {119, 0, 0}, {120, 0, 0}, {121, 0, 0}, {122, 0, 0}, {123, 0, 0}, {124, 0, 0}, {125, 0, 0}, {126, 0, 0}, {127, 0, 0}, {128, 0, 0}, {129, 0, 0}, {130, 0, 0}, {131, 0, 0}, {132, 0, 0}, {133, 0, 0}, {134, 0, 0}, {135, 0, 0}, {136, 0, 0}, {137, 0, 0}, {138, 0, 0}, {139, 0, 0}, {140, 0, 0}, {141, 0, 0}, {142, 0, 0}, {143, 0, 0}, {144, 0, 0}, {145, 0, 0}, {146, 0, 0}, {147, 0, 0}, {148, 0, 0}, {149, 0, 0}, {150, 0, 0}, {151, 0, 0}, {152, 0, 0}, {153, 0, 0}, {154, 0, 0}, {155, 0, 0}, {156, 0, 0}, {157, 0, 0}, {158, 0, 0}, {159, 0, 0}, {160, 0, 0}, {161, 0, 0}, {162, 0, 0}, {163, 0, 0}, {164, 0, 0}, {165, 0, 0}, {166, 0, 0}, {167, 0, 0}, {168, 0, 0}, {169, 0, 0}, {170, 0, 0}, {171, 0, 0}, {172, 0, 0}, {173, 0, 0}, {174, 0, 0}, {175, 0, 0}, {176, 0, 0}, {177, 0, 0}, {178, 0, 0}, {179, 0, 0}, {180, 0, 0}, {181, 0, 0}, {182, 0, 0}, {183, 0, 0}, {184, 0, 0}, {185, 0, 0}, {186, 0, 0}, {187, 0, 0}, {188, 0, 0}, {189, 0, 0}, {190, 0, 0}, {191, 0, 0}, {192, 0, 0}, {193, 0, 0}, {194, 0, 0}, {195, 0, 0}, {196, 0, 0}, {197, 0, 0}, {198, 0, 0}, {199, 0, 0}, {200, 0, 0}, {201, 0, 0}, {202, 0, 0}, {203, 0, 0}, {204, 0, 0}, {205, 0, 0}, {206, 0, 0}, {207, 0, 0}, {208, 0, 0}, {209, 0, 0}, {210, 0, 0}, {211, 0, 0}, {212, 0, 0}, {213, 0, 0}, {214, 0, 0}, {215, 0, 0}, {216, 0, 0}, {217, 0, 0}, {218, 0, 0}, {219, 0, 0}, {220, 0, 0}, {221, 0, 0}, {222, 0, 0}, {223, 0, 0}, {224, 0, 0}, {225, 0, 0}, {226, 0, 0}, {227, 0, 0}, {228, 0, 0}, {229, 0, 0}, {230, 0, 0}, {231, 0, 0}, {232, 0, 0}, {233, 0, 0}, {234, 0, 0}, {235, 0, 0}, {236, 0, 0}, {237, 0, 0}, {238, 0, 0}, {239, 0, 0}, {240, 0, 0}, {241, 0, 0}, {242, 0, 0}, {243, 0, 0}, {244, 0, 0}, {245, 0, 0}, {246, 0, 0}, {247, 0, 0}, {248, 0, 0}, {249, 0, 0}, {250, 0, 0}, {251, 0, 0}, {252, 0, 0}, {253, 0, 0}, {254, 0, 0}, {255, 0, 0}] ("Array") cluster{u8, u8, u8}[] [{0, 0, 0}, {0, 1, 0}, {0, 2, 0}, {0, 3, 0}, {0, 4, 0}, {0, 5, 0}, {0, 6, 0}, {0, 7, 0}, {0, 8, 0}, {0, 9, 0}, {0, 10, 0}, {0, 11, 0}, {0, 12, 0}, {0, 13, 0}, {0, 14, 0}, {0, 15, 0}, {0, 16, 0}, {0, 17, 0}, {0, 18, 0}, {0, 19, 0}, {0, 20, 0}, {0, 21, 0}, {0, 22, 0}, {0, 23, 0}, {0, 24, 0}, {0, 25, 0}, {0, 26, 0}, {0, 27, 0}, {0, 28, 0}, {0, 29, 0}, {0, 30, 0}, {0, 31, 0}, {0, 32, 0}, {0, 33, 0}, {0, 34, 0}, {0, 35, 0}, {0, 36, 0}, {0, 37, 0}, {0, 38, 0}, {0, 39, 0}, {0, 40, 0}, {0, 41, 0}, {0, 42, 0}, {0, 43, 0}, {0, 44, 0}, {0, 45, 0}, {0, 46, 0}, {0, 47, 0}, {0, 48, 0}, {0, 49, 0}, {0, 50, 0}, {0, 51, 0}, {0, 52, 0}, {0, 53, 0}, {0, 54, 0}, {0, 55, 0}, {0, 56, 0}, {0, 57, 0}, {0, 58, 0}, {0, 59, 0}, {0, 60, 0}, {0, 61, 0}, {0, 62, 0}, {0, 63, 0}, {0, 64, 0}, {0, 65, 0}, {0, 66, 0}, {0, 67, 0}, {0, 68, 0}, {0, 69, 0}, {0, 70, 0}, {0, 71, 0}, {0, 72, 0}, {0, 73, 0}, {0, 74, 0}, {0, 75, 0}, {0, 76, 0}, {0, 77, 0}, {0, 78, 0}, {0, 79, 0}, {0, 80, 0}, {0, 81, 0}, {0, 82, 0}, {0, 83, 0}, {0, 84, 0}, {0, 85, 0}, {0, 86, 0}, {0, 87, 0}, {0, 88, 0}, {0, 89, 0}, {0, 90, 0}, {0, 91, 0}, {0, 92, 0}, {0, 93, 0}, {0, 94, 0}, {0, 95, 0}, {0, 96, 0}, {0, 97, 0}, {0, 98, 0}, {0, 99, 0}, {0, 100, 0}, {0, 101, 0}, {0, 102, 0}, {0, 103, 0}, {0, 104, 0}, {0, 105, 0}, {0, 106, 0}, {0, 107, 0}, {0, 108, 0}, {0, 109, 0}, {0, 110, 0}, {0, 111, 0}, {0, 112, 0}, {0, 113, 0}, {0, 114, 0}, {0, 115, 0}, {0, 116, 0}, {0, 117, 0}, {0, 118, 0}, {0, 119, 0}, {0, 120, 0}, {0, 121, 0}, {0, 122, 0}, {0, 123, 0}, {0, 124, 0}, {0, 125, 0}, {0, 126, 0}, {0, 127, 0}, {0, 128, 0}, {0, 129, 0}, {0, 130, 0}, {0, 131, 0}, {0, 132, 0}, {0, 133, 0}, {0, 134, 0}, {0, 135, 0}, {0, 136, 0}, {0, 137, 0}, {0, 138, 0}, {0, 139, 0}, {0, 140, 0}, {0, 141, 0}, {0, 142, 0}, {0, 143, 0}, {0, 144, 0}, {0, 145, 0}, {0, 146, 0}, {0, 147, 0}, {0, 148, 0}, {0, 149, 0}, {0, 150, 0}, {0, 151, 0}, {0, 152, 0}, {0, 153, 0}, {0, 154, 0}, {0, 155, 0}, {0, 156, 0}, {0, 157, 0}, {0, 158, 0}, {0, 159, 0}, {0, 160, 0}, {0, 161, 0}, {0, 162, 0}, {0, 163, 0}, {0, 164, 0}, {0, 165, 0}, {0, 166, 0}, {0, 167, 0}, {0, 168, 0}, {0, 169, 0}, {0, 170, 0}, {0, 171, 0}, {0, 172, 0}, {0, 173, 0}, {0, 174, 0}, {0, 175, 0}, {0, 176, 0}, {0, 177, 0}, {0, 178, 0}, {0, 179, 0}, {0, 180, 0}, {0, 181, 0}, {0, 182, 0}, {0, 183, 0}, {0, 184, 0}, {0, 185, 0}, {0, 186, 0}, {0, 187, 0}, {0, 188, 0}, {0, 189, 0}, {0, 190, 0}, {0, 191, 0}, {0, 192, 0}, {0, 193, 0}, {0, 194, 0}, {0, 195, 0}, {0, 196, 0}, {0, 197, 0}, {0, 198, 0}, {0, 199, 0}, {0, 200, 0}, {0, 201, 0}, {0, 202, 0}, {0, 203, 0}, {0, 204, 0}, {0, 205, 0}, {0, 206, 0}, {0, 207, 0}, {0, 208, 0}, {0, 209, 0}, {0, 210, 0}, {0, 211, 0}, {0, 212, 0}, {0, 213, 0}, {0, 214, 0}, {0, 215, 0}, {0, 216, 0}, {0, 217, 0}, {0, 218, 0}, {0, 219, 0}, {0, 220, 0}, {0, 221, 0}, {0, 222, 0}, {0, 223, 0}, {0, 224, 0}, {0, 225, 0}, {0, 226, 0}, {0, 227, 0}, {0, 228, 0}, {0, 229, 0}, {0, 230, 0}, {0, 231, 0}, {0, 232, 0}, {0, 233, 0}, {0, 234, 0}, {0, 235, 0}, {0, 236, 0}, {0, 237, 0}, {0, 238, 0}, {0, 239, 0}, {0, 240, 0}, {0, 241, 0}, {0, 242, 0}, {0, 243, 0}, {0, 244, 0}, {0, 245, 0}, {0, 246, 0}, {0, 247, 0}, {0, 248, 0}, {0, 249, 0}, {0, 250, 0}, {0, 251, 0}, {0, 252, 0}, {0, 253, 0}, {0, 254, 0}, {0, 255, 0}] ("Array") cluster{u8, u8, u8}[] [{0, 0, 0}, {0, 0, 1}, {0, 0, 2}, {0, 0, 3}, {0, 0, 4}, {0, 0, 5}, {0, 0, 6}, {0, 0, 7}, {0, 0, 8}, {0, 0, 9}, {0, 0, 10}, {0, 0, 11}, {0, 0, 12}, {0, 0, 13}, {0, 0, 14}, {0, 0, 15}, {0, 0, 16}, {0, 0, 17}, {0, 0, 18}, {0, 0, 19}, {0, 0, 20}, {0, 0, 21}, {0, 0, 22}, {0, 0, 23}, {0, 0, 24}, {0, 0, 25}, {0, 0, 26}, {0, 0, 27}, {0, 0, 28}, {0, 0, 29}, {0, 0, 30}, {0, 0, 31}, {0, 0, 32}, {0, 0, 33}, {0, 0, 34}, {0, 0, 35}, {0, 0, 36}, {0, 0, 37}, {0, 0, 38}, {0, 0, 39}, {0, 0, 40}, {0, 0, 41}, {0, 0, 42}, {0, 0, 43}, {0, 0, 44}, {0, 0, 45}, {0, 0, 46}, {0, 0, 47}, {0, 0, 48}, {0, 0, 49}, {0, 0, 50}, {0, 0, 51}, {0, 0, 52}, {0, 0, 53}, {0, 0, 54}, {0, 0, 55}, {0, 0, 56}, {0, 0, 57}, {0, 0, 58}, {0, 0, 59}, {0, 0, 60}, {0, 0, 61}, {0, 0, 62}, {0, 0, 63}, {0, 0, 64}, {0, 0, 65}, {0, 0, 66}, {0, 0, 67}, {0, 0, 68}, {0, 0, 69}, {0, 0, 70}, {0, 0, 71}, {0, 0, 72}, {0, 0, 73}, {0, 0, 74}, {0, 0, 75}, {0, 0, 76}, {0, 0, 77}, {0, 0, 78}, {0, 0, 79}, {0, 0, 80}, {0, 0, 81}, {0, 0, 82}, {0, 0, 83}, {0, 0, 84}, {0, 0, 85}, {0, 0, 86}, {0, 0, 87}, {0, 0, 88}, {0, 0, 89}, {0, 0, 90}, {0, 0, 91}, {0, 0, 92}, {0, 0, 93}, {0, 0, 94}, {0, 0, 95}, {0, 0, 96}, {0, 0, 97}, {0, 0, 98}, {0, 0, 99}, {0, 0, 100}, {0, 0, 101}, {0, 0, 102}, {0, 0, 103}, {0, 0, 104}, {0, 0, 105}, {0, 0, 106}, {0, 0, 107}, {0, 0, 108}, {0, 0, 109}, {0, 0, 110}, {0, 0, 111}, {0, 0, 112}, {0, 0, 113}, {0, 0, 114}, {0, 0, 115}, {0, 0, 116}, {0, 0, 117}, {0, 0, 118}, {0, 0, 119}, {0, 0, 120}, {0, 0, 121}, {0, 0, 122}, {0, 0, 123}, {0, 0, 124}, {0, 0, 125}, {0, 0, 126}, {0, 0, 127}, {0, 0, 128}, {0, 0, 129}, {0, 0, 130}, {0, 0, 131}, {0, 0, 132}, {0, 0, 133}, {0, 0, 134}, {0, 0, 135}, {0, 0, 136}, {0, 0, 137}, {0, 0, 138}, {0, 0, 139}, {0, 0, 140}, {0, 0, 141}, {0, 0, 142}, {0, 0, 143}, {0, 0, 144}, {0, 0, 145}, {0, 0, 146}, {0, 0, 147}, {0, 0, 148}, {0, 0, 149}, {0, 0, 150}, {0, 0, 151}, {0, 0, 152}, {0, 0, 153}, {0, 0, 154}, {0, 0, 155}, {0, 0, 156}, {0, 0, 157}, {0, 0, 158}, {0, 0, 159}, {0, 0, 160}, {0, 0, 161}, {0, 0, 162}, {0, 0, 163}, {0, 0, 164}, {0, 0, 165}, {0, 0, 166}, {0, 0, 167}, {0, 0, 168}, {0, 0, 169}, {0, 0, 170}, {0, 0, 171}, {0, 0, 172}, {0, 0, 173}, {0, 0, 174}, {0, 0, 175}, {0, 0, 176}, {0, 0, 177}, {0, 0, 178}, {0, 0, 179}, {0, 0, 180}, {0, 0, 181}, {0, 0, 182}, {0, 0, 183}, {0, 0, 184}, {0, 0, 185}, {0, 0, 186}, {0, 0, 187}, {0, 0, 188}, {0, 0, 189}, {0, 0, 190}, {0, 0, 191}, {0, 0, 192}, {0, 0, 193}, {0, 0, 194}, {0, 0, 195}, {0, 0, 196}, {0, 0, 197}, {0, 0, 198}, {0, 0, 199}, {0, 0, 200}, {0, 0, 201}, {0, 0, 202}, {0, 0, 203}, {0, 0, 204}, {0, 0, 205}, {0, 0, 206}, {0, 0, 207}, {0, 0, 208}, {0, 0, 209}, {0, 0, 210}, {0, 0, 211}, {0, 0, 212}, {0, 0, 213}, {0, 0, 214}, {0, 0, 215}, {0, 0, 216}, {0, 0, 217}, {0, 0, 218}, {0, 0, 219}, {0, 0, 220}, {0, 0, 221}, {0, 0, 222}, {0, 0, 223}, {0, 0, 224}, {0, 0, 225}, {0, 0, 226}, {0, 0, 227}, {0, 0, 228}, {0, 0, 229}, {0, 0, 230}, {0, 0, 231}, {0, 0, 232}, {0, 0, 233}, {0, 0, 234}, {0, 0, 235}, {0, 0, 236}, {0, 0, 237}, {0, 0, 238}, {0, 0, 239}, {0, 0, 240}, {0, 0, 241}, {0, 0, 242}, {0, 0, 243}, {0, 0, 244}, {0, 0, 245}, {0, 0, 246}, {0, 0, 247}, {0, 0, 248}, {0, 0, 249}, {0, 0, 250}, {0, 0, 251}, {0, 0, 252}, {0, 0, 253}, {0, 0, 254}, {0, 0, 255}] ("Array") cluster{u8, u8, u8}[] [{0, 0, 0}, {0, 1, 1}, {0, 2, 2}, {0, 3, 3}, {0, 4, 4}, {0, 5, 5}, {0, 6, 6}, {0, 7, 7}, {0, 8, 8}, {0, 9, 9}, {0, 10, 10}, {0, 11, 11}, {0, 12, 12}, {0, 13, 13}, {0, 14, 14}, {0, 15, 15}, {0, 16, 16}, {0, 17, 17}, {0, 18, 18}, {0, 19, 19}, {0, 20, 20}, {0, 21, 21}, {0, 22, 22}, {0, 23, 23}, {0, 24, 24}, {0, 25, 25}, {0, 26, 26}, {0, 27, 27}, {0, 28, 28}, {0, 29, 29}, {0, 30, 30}, {0, 31, 31}, {0, 32, 32}, {0, 33, 33}, {0, 34, 34}, {0, 35, 35}, {0, 36, 36}, {0, 37, 37}, {0, 38, 38}, {0, 39, 39}, {0, 40, 40}, {0, 41, 41}, {0, 42, 42}, {0, 43, 43}, {0, 44, 44}, {0, 45, 45}, {0, 46, 46}, {0, 47, 47}, {0, 48, 48}, {0, 49, 49}, {0, 50, 50}, {0, 51, 51}, {0, 52, 52}, {0, 53, 53}, {0, 54, 54}, {0, 55, 55}, {0, 56, 56}, {0, 57, 57}, {0, 58, 58}, {0, 59, 59}, {0, 60, 60}, {0, 61, 61}, {0, 62, 62}, {0, 63, 63}, {0, 64, 64}, {0, 65, 65}, {0, 66, 66}, {0, 67, 67}, {0, 68, 68}, {0, 69, 69}, {0, 70, 70}, {0, 71, 71}, {0, 72, 72}, {0, 73, 73}, {0, 74, 74}, {0, 75, 75}, {0, 76, 76}, {0, 77, 77}, {0, 78, 78}, {0, 79, 79}, {0, 80, 80}, {0, 81, 81}, {0, 82, 82}, {0, 83, 83}, {0, 84, 84}, {0, 85, 85}, {0, 86, 86}, {0, 87, 87}, {0, 88, 88}, {0, 89, 89}, {0, 90, 90}, {0, 91, 91}, {0, 92, 92}, {0, 93, 93}, {0, 94, 94}, {0, 95, 95}, {0, 96, 96}, {0, 97, 97}, {0, 98, 98}, {0, 99, 99}, {0, 100, 100}, {0, 101, 101}, {0, 102, 102}, {0, 103, 103}, {0, 104, 104}, {0, 105, 105}, {0, 106, 106}, {0, 107, 107}, {0, 108, 108}, {0, 109, 109}, {0, 110, 110}, {0, 111, 111}, {0, 112, 112}, {0, 113, 113}, {0, 114, 114}, {0, 115, 115}, {0, 116, 116}, {0, 117, 117}, {0, 118, 118}, {0, 119, 119}, {0, 120, 120}, {0, 121, 121}, {0, 122, 122}, {0, 123, 123}, {0, 124, 124}, {0, 125, 125}, {0, 126, 126}, {0, 127, 127}, {0, 128, 128}, {0, 129, 129}, {0, 130, 130}, {0, 131, 131}, {0, 132, 132}, {0, 133, 133}, {0, 134, 134}, {0, 135, 135}, {0, 136, 136}, {0, 137, 137}, {0, 138, 138}, {0, 139, 139}, {0, 140, 140}, {0, 141, 141}, {0, 142, 142}, {0, 143, 143}, {0, 144, 144}, {0, 145, 145}, {0, 146, 146}, {0, 147, 147}, {0, 148, 148}, {0, 149, 149}, {0, 150, 150}, {0, 151, 151}, {0, 152, 152}, {0, 153, 153}, {0, 154, 154}, {0, 155, 155}, {0, 156, 156}, {0, 157, 157}, {0, 158, 158}, {0, 159, 159}, {0, 160, 160}, {0, 161, 161}, {0, 162, 162}, {0, 163, 163}, {0, 164, 164}, {0, 165, 165}, {0, 166, 166}, {0, 167, 167}, {0, 168, 168}, {0, 169, 169}, {0, 170, 170}, {0, 171, 171}, {0, 172, 172}, {0, 173, 173}, {0, 174, 174}, {0, 175, 175}, {0, 176, 176}, {0, 177, 177}, {0, 178, 178}, {0, 179, 179}, {0, 180, 180}, {0, 181, 181}, {0, 182, 182}, {0, 183, 183}, {0, 184, 184}, {0, 185, 185}, {0, 186, 186}, {0, 187, 187}, {0, 188, 188}, {0, 189, 189}, {0, 190, 190}, {0, 191, 191}, {0, 192, 192}, {0, 193, 193}, {0, 194, 194}, {0, 195, 195}, {0, 196, 196}, {0, 197, 197}, {0, 198, 198}, {0, 199, 199}, {0, 200, 200}, {0, 201, 201}, {0, 202, 202}, {0, 203, 203}, {0, 204, 204}, {0, 205, 205}, {0, 206, 206}, {0, 207, 207}, {0, 208, 208}, {0, 209, 209}, {0, 210, 210}, {0, 211, 211}, {0, 212, 212}, {0, 213, 213}, {0, 214, 214}, {0, 215, 215}, {0, 216, 216}, {0, 217, 217}, {0, 218, 218}, {0, 219, 219}, {0, 220, 220}, {0, 221, 221}, {0, 222, 222}, {0, 223, 223}, {0, 224, 224}, {0, 225, 225}, {0, 226, 226}, {0, 227, 227}, {0, 228, 228}, {0, 229, 229}, {0, 230, 230}, {0, 231, 231}, {0, 232, 232}, {0, 233, 233}, {0, 234, 234}, {0, 235, 235}, {0, 236, 236}, {0, 237, 237}, {0, 238, 238}, {0, 239, 239}, {0, 240, 240}, {0, 241, 241}, {0, 242, 242}, {0, 243, 243}, {0, 244, 244}, {0, 245, 245}, {0, 246, 246}, {0, 247, 247}, {0, 248, 248}, {0, 249, 249}, {0, 250, 250}, {0, 251, 251}, {0, 252, 252}, {0, 253, 253}, {0, 254, 254}, {0, 255, 255}] ("Array") cluster{u8, u8, u8}[] [{0, 0, 0}, {1, 0, 1}, {2, 0, 2}, {3, 0, 3}, {4, 0, 4}, {5, 0, 5}, {6, 0, 6}, {7, 0, 7}, {8, 0, 8}, {9, 0, 9}, {10, 0, 10}, {11, 0, 11}, {12, 0, 12}, {13, 0, 13}, {14, 0, 14}, {15, 0, 15}, {16, 0, 16}, {17, 0, 17}, {18, 0, 18}, {19, 0, 19}, {20, 0, 20}, {21, 0, 21}, {22, 0, 22}, {23, 0, 23}, {24, 0, 24}, {25, 0, 25}, {26, 0, 26}, {27, 0, 27}, {28, 0, 28}, {29, 0, 29}, {30, 0, 30}, {31, 0, 31}, {32, 0, 32}, {33, 0, 33}, {34, 0, 34}, {35, 0, 35}, {36, 0, 36}, {37, 0, 37}, {38, 0, 38}, {39, 0, 39}, {40, 0, 40}, {41, 0, 41}, {42, 0, 42}, {43, 0, 43}, {44, 0, 44}, {45, 0, 45}, {46, 0, 46}, {47, 0, 47}, {48, 0, 48}, {49, 0, 49}, {50, 0, 50}, {51, 0, 51}, {52, 0, 52}, {53, 0, 53}, {54, 0, 54}, {55, 0, 55}, {56, 0, 56}, {57, 0, 57}, {58, 0, 58}, {59, 0, 59}, {60, 0, 60}, {61, 0, 61}, {62, 0, 62}, {63, 0, 63}, {64, 0, 64}, {65, 0, 65}, {66, 0, 66}, {67, 0, 67}, {68, 0, 68}, {69, 0, 69}, {70, 0, 70}, {71, 0, 71}, {72, 0, 72}, {73, 0, 73}, {74, 0, 74}, {75, 0, 75}, {76, 0, 76}, {77, 0, 77}, {78, 0, 78}, {79, 0, 79}, {80, 0, 80}, {81, 0, 81}, {82, 0, 82}, {83, 0, 83}, {84, 0, 84}, {85, 0, 85}, {86, 0, 86}, {87, 0, 87}, {88, 0, 88}, {89, 0, 89}, {90, 0, 90}, {91, 0, 91}, {92, 0, 92}, {93, 0, 93}, {94, 0, 94}, {95, 0, 95}, {96, 0, 96}, {97, 0, 97}, {98, 0, 98}, {99, 0, 99}, {100, 0, 100}, {101, 0, 101}, {102, 0, 102}, {103, 0, 103}, {104, 0, 104}, {105, 0, 105}, {106, 0, 106}, {107, 0, 107}, {108, 0, 108}, {109, 0, 109}, {110, 0, 110}, {111, 0, 111}, {112, 0, 112}, {113, 0, 113}, {114, 0, 114}, {115, 0, 115}, {116, 0, 116}, {117, 0, 117}, {118, 0, 118}, {119, 0, 119}, {120, 0, 120}, {121, 0, 121}, {122, 0, 122}, {123, 0, 123}, {124, 0, 124}, {125, 0, 125}, {126, 0, 126}, {127, 0, 127}, {128, 0, 128}, {129, 0, 129}, {130, 0, 130}, {131, 0, 131}, {132, 0, 132}, {133, 0, 133}, {134, 0, 134}, {135, 0, 135}, {136, 0, 136}, {137, 0, 137}, {138, 0, 138}, {139, 0, 139}, {140, 0, 140}, {141, 0, 141}, {142, 0, 142}, {143, 0, 143}, {144, 0, 144}, {145, 0, 145}, {146, 0, 146}, {147, 0, 147}, {148, 0, 148}, {149, 0, 149}, {150, 0, 150}, {151, 0, 151}, {152, 0, 152}, {153, 0, 153}, {154, 0, 154}, {155, 0, 155}, {156, 0, 156}, {157, 0, 157}, {158, 0, 158}, {159, 0, 159}, {160, 0, 160}, {161, 0, 161}, {162, 0, 162}, {163, 0, 163}, {164, 0, 164}, {165, 0, 165}, {166, 0, 166}, {167, 0, 167}, {168, 0, 168}, {169, 0, 169}, {170, 0, 170}, {171, 0, 171}, {172, 0, 172}, {173, 0, 173}, {174, 0, 174}, {175, 0, 175}, {176, 0, 176}, {177, 0, 177}, {178, 0, 178}, {179, 0, 179}, {180, 0, 180}, {181, 0, 181}, {182, 0, 182}, {183, 0, 183}, {184, 0, 184}, {185, 0, 185}, {186, 0, 186}, {187, 0, 187}, {188, 0, 188}, {189, 0, 189}, {190, 0, 190}, {191, 0, 191}, {192, 0, 192}, {193, 0, 193}, {194, 0, 194}, {195, 0, 195}, {196, 0, 196}, {197, 0, 197}, {198, 0, 198}, {199, 0, 199}, {200, 0, 200}, {201, 0, 201}, {202, 0, 202}, {203, 0, 203}, {204, 0, 204}, {205, 0, 205}, {206, 0, 206}, {207, 0, 207}, {208, 0, 208}, {209, 0, 209}, {210, 0, 210}, {211, 0, 211}, {212, 0, 212}, {213, 0, 213}, {214, 0, 214}, {215, 0, 215}, {216, 0, 216}, {217, 0, 217}, {218, 0, 218}, {219, 0, 219}, {220, 0, 220}, {221, 0, 221}, {222, 0, 222}, {223, 0, 223}, {224, 0, 224}, {225, 0, 225}, {226, 0, 226}, {227, 0, 227}, {228, 0, 228}, {229, 0, 229}, {230, 0, 230}, {231, 0, 231}, {232, 0, 232}, {233, 0, 233}, {234, 0, 234}, {235, 0, 235}, {236, 0, 236}, {237, 0, 237}, {238, 0, 238}, {239, 0, 239}, {240, 0, 240}, {241, 0, 241}, {242, 0, 242}, {243, 0, 243}, {244, 0, 244}, {245, 0, 245}, {246, 0, 246}, {247, 0, 247}, {248, 0, 248}, {249, 0, 249}, {250, 0, 250}, {251, 0, 251}, {252, 0, 252}, {253, 0, 253}, {254, 0, 254}, {255, 0, 255}] ("Array") cluster{u8, u8, u8}[] [{0, 0, 0}, {1, 1, 0}, {2, 2, 0}, {3, 3, 0}, {4, 4, 0}, {5, 5, 0}, {6, 6, 0}, {7, 7, 0}, {8, 8, 0}, {9, 9, 0}, {10, 10, 0}, {11, 11, 0}, {12, 12, 0}, {13, 13, 0}, {14, 14, 0}, {15, 15, 0}, {16, 16, 0}, {17, 17, 0}, {18, 18, 0}, {19, 19, 0}, {20, 20, 0}, {21, 21, 0}, {22, 22, 0}, {23, 23, 0}, {24, 24, 0}, {25, 25, 0}, {26, 26, 0}, {27, 27, 0}, {28, 28, 0}, {29, 29, 0}, {30, 30, 0}, {31, 31, 0}, {32, 32, 0}, {33, 33, 0}, {34, 34, 0}, {35, 35, 0}, {36, 36, 0}, {37, 37, 0}, {38, 38, 0}, {39, 39, 0}, {40, 40, 0}, {41, 41, 0}, {42, 42, 0}, {43, 43, 0}, {44, 44, 0}, {45, 45, 0}, {46, 46, 0}, {47, 47, 0}, {48, 48, 0}, {49, 49, 0}, {50, 50, 0}, {51, 51, 0}, {52, 52, 0}, {53, 53, 0}, {54, 54, 0}, {55, 55, 0}, {56, 56, 0}, {57, 57, 0}, {58, 58, 0}, {59, 59, 0}, {60, 60, 0}, {61, 61, 0}, {62, 62, 0}, {63, 63, 0}, {64, 64, 0}, {65, 65, 0}, {66, 66, 0}, {67, 67, 0}, {68, 68, 0}, {69, 69, 0}, {70, 70, 0}, {71, 71, 0}, {72, 72, 0}, {73, 73, 0}, {74, 74, 0}, {75, 75, 0}, {76, 76, 0}, {77, 77, 0}, {78, 78, 0}, {79, 79, 0}, {80, 80, 0}, {81, 81, 0}, {82, 82, 0}, {83, 83, 0}, {84, 84, 0}, {85, 85, 0}, {86, 86, 0}, {87, 87, 0}, {88, 88, 0}, {89, 89, 0}, {90, 90, 0}, {91, 91, 0}, {92, 92, 0}, {93, 93, 0}, {94, 94, 0}, {95, 95, 0}, {96, 96, 0}, {97, 97, 0}, {98, 98, 0}, {99, 99, 0}, {100, 100, 0}, {101, 101, 0}, {102, 102, 0}, {103, 103, 0}, {104, 104, 0}, {105, 105, 0}, {106, 106, 0}, {107, 107, 0}, {108, 108, 0}, {109, 109, 0}, {110, 110, 0}, {111, 111, 0}, {112, 112, 0}, {113, 113, 0}, {114, 114, 0}, {115, 115, 0}, {116, 116, 0}, {117, 117, 0}, {118, 118, 0}, {119, 119, 0}, {120, 120, 0}, {121, 121, 0}, {122, 122, 0}, {123, 123, 0}, {124, 124, 0}, {125, 125, 0}, {126, 126, 0}, {127, 127, 0}, {128, 128, 0}, {129, 129, 0}, {130, 130, 0}, {131, 131, 0}, {132, 132, 0}, {133, 133, 0}, {134, 134, 0}, {135, 135, 0}, {136, 136, 0}, {137, 137, 0}, {138, 138, 0}, {139, 139, 0}, {140, 140, 0}, {141, 141, 0}, {142, 142, 0}, {143, 143, 0}, {144, 144, 0}, {145, 145, 0}, {146, 146, 0}, {147, 147, 0}, {148, 148, 0}, {149, 149, 0}, {150, 150, 0}, {151, 151, 0}, {152, 152, 0}, {153, 153, 0}, {154, 154, 0}, {155, 155, 0}, {156, 156, 0}, {157, 157, 0}, {158, 158, 0}, {159, 159, 0}, {160, 160, 0}, {161, 161, 0}, {162, 162, 0}, {163, 163, 0}, {164, 164, 0}, {165, 165, 0}, {166, 166, 0}, {167, 167, 0}, {168, 168, 0}, {169, 169, 0}, {170, 170, 0}, {171, 171, 0}, {172, 172, 0}, {173, 173, 0}, {174, 174, 0}, {175, 175, 0}, {176, 176, 0}, {177, 177, 0}, {178, 178, 0}, {179, 179, 0}, {180, 180, 0}, {181, 181, 0}, {182, 182, 0}, {183, 183, 0}, {184, 184, 0}, {185, 185, 0}, {186, 186, 0}, {187, 187, 0}, {188, 188, 0}, {189, 189, 0}, {190, 190, 0}, {191, 191, 0}, {192, 192, 0}, {193, 193, 0}, {194, 194, 0}, {195, 195, 0}, {196, 196, 0}, {197, 197, 0}, {198, 198, 0}, {199, 199, 0}, {200, 200, 0}, {201, 201, 0}, {202, 202, 0}, {203, 203, 0}, {204, 204, 0}, {205, 205, 0}, {206, 206, 0}, {207, 207, 0}, {208, 208, 0}, {209, 209, 0}, {210, 210, 0}, {211, 211, 0}, {212, 212, 0}, {213, 213, 0}, {214, 214, 0}, {215, 215, 0}, {216, 216, 0}, {217, 217, 0}, {218, 218, 0}, {219, 219, 0}, {220, 220, 0}, {221, 221, 0}, {222, 222, 0}, {223, 223, 0}, {224, 224, 0}, {225, 225, 0}, {226, 226, 0}, {227, 227, 0}, {228, 228, 0}, {229, 229, 0}, {230, 230, 0}, {231, 231, 0}, {232, 232, 0}, {233, 233, 0}, {234, 234, 0}, {235, 235, 0}, {236, 236, 0}, {237, 237, 0}, {238, 238, 0}, {239, 239, 0}, {240, 240, 0}, {241, 241, 0}, {242, 242, 0}, {243, 243, 0}, {244, 244, 0}, {245, 245, 0}, {246, 246, 0}, {247, 247, 0}, {248, 248, 0}, {249, 249, 0}, {250, 250, 0}, {251, 251, 0}, {252, 252, 0}, {253, 253, 0}, {254, 254, 0}, {255, 255, 0}] ("Array") cluster{u8, u8, u8}[] [{0, 0, 0}, {2, 0, 0}, {3, 0, 0}, {4, 0, 0}, {6, 0, 0}, {8, 0, 0}, {9, 0, 0}, {10, 0, 0}, {12, 0, 0}, {14, 0, 0}, {15, 0, 0}, {16, 0, 0}, {18, 0, 0}, {20, 0, 0}, {21, 0, 0}, {22, 0, 0}, {24, 0, 0}, {26, 0, 0}, {27, 0, 0}, {28, 0, 0}, {30, 0, 0}, {32, 0, 0}, {33, 0, 0}, {34, 0, 0}, {36, 0, 0}, {38, 0, 0}, {39, 0, 0}, {40, 0, 0}, {42, 0, 0}, {44, 0, 0}, {45, 0, 0}, {46, 0, 0}, {48, 0, 0}, {50, 0, 0}, {51, 0, 0}, {52, 0, 0}, {54, 0, 0}, {56, 0, 0}, {57, 0, 0}, {58, 0, 0}, {60, 0, 0}, {62, 0, 0}, {63, 0, 0}, {64, 0, 0}, {66, 0, 0}, {68, 0, 0}, {69, 0, 0}, {70, 0, 0}, {72, 0, 0}, {74, 0, 0}, {75, 0, 0}, {76, 0, 0}, {78, 0, 0}, {80, 0, 0}, {81, 0, 0}, {82, 0, 0}, {84, 0, 0}, {86, 0, 0}, {87, 0, 0}, {88, 0, 0}, {90, 0, 0}, {92, 0, 0}, {93, 0, 0}, {94, 0, 0}, {96, 0, 0}, {98, 0, 0}, {99, 0, 0}, {100, 0, 0}, {102, 0, 0}, {104, 0, 0}, {105, 0, 0}, {106, 0, 0}, {108, 0, 0}, {110, 0, 0}, {111, 0, 0}, {112, 0, 0}, {114, 0, 0}, {116, 0, 0}, {117, 0, 0}, {118, 0, 0}, {120, 0, 0}, {122, 0, 0}, {123, 0, 0}, {124, 0, 0}, {126, 0, 0}, {128, 0, 0}, {129, 0, 0}, {130, 0, 0}, {132, 0, 0}, {134, 0, 0}, {135, 0, 0}, {136, 0, 0}, {138, 0, 0}, {140, 0, 0}, {141, 0, 0}, {142, 0, 0}, {144, 0, 0}, {146, 0, 0}, {147, 0, 0}, {148, 0, 0}, {150, 0, 0}, {152, 0, 0}, {153, 0, 0}, {154, 0, 0}, {156, 0, 0}, {158, 0, 0}, {159, 0, 0}, {160, 0, 0}, {162, 0, 0}, {164, 0, 0}, {165, 0, 0}, {166, 0, 0}, {168, 0, 0}, {170, 0, 0}, {171, 0, 0}, {172, 0, 0}, {174, 0, 0}, {176, 0, 0}, {177, 0, 0}, {178, 0, 0}, {180, 0, 0}, {182, 0, 0}, {183, 0, 0}, {184, 0, 0}, {186, 0, 0}, {188, 0, 0}, {189, 0, 0}, {190, 0, 0}, {192, 0, 0}, {194, 0, 0}, {195, 0, 0}, {196, 0, 0}, {198, 0, 0}, {200, 0, 0}, {201, 0, 0}, {202, 0, 0}, {204, 0, 0}, {206, 0, 0}, {207, 0, 0}, {208, 0, 0}, {210, 0, 0}, {212, 0, 0}, {213, 0, 0}, {214, 0, 0}, {216, 0, 0}, {218, 0, 0}, {219, 0, 0}, {220, 0, 0}, {222, 0, 0}, {224, 0, 0}, {225, 0, 0}, {226, 0, 0}, {228, 0, 0}, {230, 0, 0}, {231, 0, 0}, {232, 0, 0}, {234, 0, 0}, {236, 0, 0}, {237, 0, 0}, {238, 0, 0}, {240, 0, 0}, {242, 0, 0}, {243, 0, 0}, {244, 0, 0}, {246, 0, 0}, {248, 0, 0}, {249, 0, 0}, {250, 0, 0}, {252, 0, 0}, {254, 0, 0}, {255, 0, 0}, {255, 3, 3}, {255, 7, 6}, {255, 10, 9}, {255, 14, 12}, {255, 17, 15}, {255, 20, 18}, {255, 24, 21}, {255, 27, 24}, {255, 31, 27}, {255, 34, 30}, {255, 37, 33}, {255, 41, 36}, {255, 44, 39}, {255, 48, 42}, {255, 51, 45}, {255, 54, 48}, {255, 58, 51}, {255, 61, 54}, {255, 65, 57}, {255, 68, 60}, {255, 71, 63}, {255, 75, 66}, {255, 78, 69}, {255, 82, 72}, {255, 85, 75}, {255, 88, 78}, {255, 92, 81}, {255, 95, 84}, {255, 99, 87}, {255, 102, 90}, {255, 105, 93}, {255, 109, 96}, {255, 112, 99}, {255, 116, 102}, {255, 119, 105}, {255, 122, 108}, {255, 126, 111}, {255, 129, 113}, {255, 133, 116}, {255, 136, 119}, {255, 139, 122}, {255, 143, 125}, {255, 146, 128}, {255, 150, 131}, {255, 153, 134}, {255, 156, 137}, {255, 160, 140}, {255, 163, 143}, {255, 167, 146}, {255, 170, 149}, {255, 173, 152}, {255, 177, 155}, {255, 180, 158}, {255, 184, 161}, {255, 187, 164}, {255, 190, 167}, {255, 194, 170}, {255, 197, 173}, {255, 201, 176}, {255, 204, 179}, {255, 207, 182}, {255, 211, 185}, {255, 214, 188}, {255, 218, 191}, {255, 221, 194}, {255, 224, 197}, {255, 228, 200}, {255, 231, 203}, {255, 235, 206}, {255, 238, 209}, {255, 241, 212}, {255, 245, 215}, {255, 248, 218}, {255, 252, 221}, {255, 255, 224}, {255, 255, 227}, {255, 255, 230}, {255, 255, 234}, {255, 255, 237}, {255, 255, 240}, {254, 254, 242}, {253, 253, 244}, {252, 252, 246}, {251, 251, 248}, {250, 250, 250}] ("Array 2") cluster{u8, u8, u8}[] [{0, 0, 0}, {0, 2, 0}, {0, 3, 0}, {0, 4, 0}, {0, 6, 0}, {0, 8, 0}, {0, 9, 0}, {0, 10, 0}, {0, 12, 0}, {0, 14, 0}, {0, 15, 0}, {0, 16, 0}, {0, 18, 0}, {0, 20, 0}, {0, 21, 0}, {0, 22, 0}, {0, 24, 0}, {0, 26, 0}, {0, 27, 0}, {0, 28, 0}, {0, 30, 0}, {0, 32, 0}, {0, 33, 0}, {0, 34, 0}, {0, 36, 0}, {0, 38, 0}, {0, 39, 0}, {0, 40, 0}, {0, 42, 0}, {0, 44, 0}, {0, 45, 0}, {0, 46, 0}, {0, 48, 0}, {0, 50, 0}, {0, 51, 0}, {0, 52, 0}, {0, 54, 0}, {0, 56, 0}, {0, 57, 0}, {0, 58, 0}, {0, 60, 0}, {0, 62, 0}, {0, 63, 0}, {0, 64, 0}, {0, 66, 0}, {0, 68, 0}, {0, 69, 0}, {0, 70, 0}, {0, 72, 0}, {0, 74, 0}, {0, 75, 0}, {0, 76, 0}, {0, 78, 0}, {0, 80, 0}, {0, 81, 0}, {0, 82, 0}, {0, 84, 0}, {0, 86, 0}, {0, 87, 0}, {0, 88, 0}, {0, 90, 0}, {0, 92, 0}, {0, 93, 0}, {0, 94, 0}, {0, 96, 0}, {0, 98, 0}, {0, 99, 0}, {0, 100, 0}, {0, 102, 0}, {0, 104, 0}, {0, 105, 0}, {0, 106, 0}, {0, 108, 0}, {0, 110, 0}, {0, 111, 0}, {0, 112, 0}, {0, 114, 0}, {0, 116, 0}, {0, 117, 0}, {0, 118, 0}, {0, 120, 0}, {0, 122, 0}, {0, 123, 0}, {0, 124, 0}, {0, 126, 0}, {0, 128, 0}, {0, 129, 0}, {0, 130, 0}, {0, 132, 0}, {0, 134, 0}, {0, 135, 0}, {0, 136, 0}, {0, 138, 0}, {0, 140, 0}, {0, 141, 0}, {0, 142, 0}, {0, 144, 0}, {0, 146, 0}, {0, 147, 0}, {0, 148, 0}, {0, 150, 0}, {0, 152, 0}, {0, 153, 0}, {0, 154, 0}, {0, 156, 0}, {0, 158, 0}, {0, 159, 0}, {0, 160, 0}, {0, 162, 0}, {0, 164, 0}, {0, 165, 0}, {0, 166, 0}, {0, 168, 0}, {0, 170, 0}, {0, 171, 0}, {0, 172, 0}, {0, 174, 0}, {0, 176, 0}, {0, 177, 0}, {0, 178, 0}, {0, 180, 0}, {0, 182, 0}, {0, 183, 0}, {0, 184, 0}, {0, 186, 0}, {0, 188, 0}, {0, 189, 0}, {0, 190, 0}, {0, 192, 0}, {0, 194, 0}, {0, 195, 0}, {0, 196, 0}, {0, 198, 0}, {0, 200, 0}, {0, 201, 0}, {0, 202, 0}, {0, 204, 0}, {0, 206, 0}, {0, 207, 0}, {0, 208, 0}, {0, 210, 0}, {0, 212, 0}, {0, 213, 0}, {0, 214, 0}, {0, 216, 0}, {0, 218, 0}, {0, 219, 0}, {0, 220, 0}, {0, 222, 0}, {0, 224, 0}, {0, 225, 0}, {0, 226, 0}, {0, 228, 0}, {0, 230, 0}, {0, 231, 0}, {0, 232, 0}, {0, 234, 0}, {0, 236, 0}, {0, 237, 0}, {0, 238, 0}, {0, 240, 0}, {0, 242, 0}, {0, 243, 0}, {0, 244, 0}, {0, 246, 0}, {0, 248, 0}, {0, 249, 0}, {0, 250, 0}, {0, 252, 0}, {0, 254, 0}, {0, 255, 0}, {3, 255, 3}, {7, 255, 6}, {10, 255, 9}, {14, 255, 12}, {17, 255, 15}, {20, 255, 18}, {24, 255, 21}, {27, 255, 24}, {31, 255, 27}, {34, 255, 30}, {37, 255, 33}, {41, 255, 36}, {44, 255, 39}, {48, 255, 42}, {51, 255, 45}, {54, 255, 48}, {58, 255, 51}, {61, 255, 54}, {65, 255, 57}, {68, 255, 60}, {71, 255, 63}, {75, 255, 66}, {78, 255, 69}, {82, 255, 72}, {85, 255, 75}, {88, 255, 78}, {92, 255, 81}, {95, 255, 84}, {99, 255, 87}, {102, 255, 90}, {105, 255, 93}, {109, 255, 96}, {112, 255, 99}, {116, 255, 102}, {119, 255, 105}, {122, 255, 108}, {126, 255, 111}, {129, 255, 113}, {133, 255, 116}, {136, 255, 119}, {139, 255, 122}, {143, 255, 125}, {146, 255, 128}, {150, 255, 131}, {153, 255, 134}, {156, 255, 137}, {160, 255, 140}, {163, 255, 143}, {167, 255, 146}, {170, 255, 149}, {173, 255, 152}, {177, 255, 155}, {180, 255, 158}, {184, 255, 161}, {187, 255, 164}, {190, 255, 167}, {194, 255, 170}, {197, 255, 173}, {201, 255, 176}, {204, 255, 179}, {207, 255, 182}, {211, 255, 185}, {214, 255, 188}, {218, 255, 191}, {221, 255, 194}, {224, 255, 197}, {228, 255, 200}, {231, 255, 203}, {235, 255, 206}, {238, 255, 209}, {241, 255, 212}, {245, 255, 215}, {248, 255, 218}, {252, 255, 221}, {255, 255, 224}, {255, 255, 227}, {255, 255, 230}, {255, 255, 234}, {255, 255, 237}, {255, 255, 240}, {254, 254, 242}, {253, 253, 244}, {252, 252, 246}, {251, 251, 248}, {250, 250, 250}] ("Array 2") cluster{u8, u8, u8}[] [{0, 0, 0}, {0, 0, 2}, {0, 0, 3}, {0, 0, 4}, {0, 0, 6}, {0, 0, 8}, {0, 0, 9}, {0, 0, 10}, {0, 0, 12}, {0, 0, 14}, {0, 0, 15}, {0, 0, 16}, {0, 0, 18}, {0, 0, 20}, {0, 0, 21}, {0, 0, 22}, {0, 0, 24}, {0, 0, 26}, {0, 0, 27}, {0, 0, 28}, {0, 0, 30}, {0, 0, 32}, {0, 0, 33}, {0, 0, 34}, {0, 0, 36}, {0, 0, 38}, {0, 0, 39}, {0, 0, 40}, {0, 0, 42}, {0, 0, 44}, {0, 0, 45}, {0, 0, 46}, {0, 0, 48}, {0, 0, 50}, {0, 0, 51}, {0, 0, 52}, {0, 0, 54}, {0, 0, 56}, {0, 0, 57}, {0, 0, 58}, {0, 0, 60}, {0, 0, 62}, {0, 0, 63}, {0, 0, 64}, {0, 0, 66}, {0, 0, 68}, {0, 0, 69}, {0, 0, 70}, {0, 0, 72}, {0, 0, 74}, {0, 0, 75}, {0, 0, 76}, {0, 0, 78}, {0, 0, 80}, {0, 0, 81}, {0, 0, 82}, {0, 0, 84}, {0, 0, 86}, {0, 0, 87}, {0, 0, 88}, {0, 0, 90}, {0, 0, 92}, {0, 0, 93}, {0, 0, 94}, {0, 0, 96}, {0, 0, 98}, {0, 0, 99}, {0, 0, 100}, {0, 0, 102}, {0, 0, 104}, {0, 0, 105}, {0, 0, 106}, {0, 0, 108}, {0, 0, 110}, {0, 0, 111}, {0, 0, 112}, {0, 0, 114}, {0, 0, 116}, {0, 0, 117}, {0, 0, 118}, {0, 0, 120}, {0, 0, 122}, {0, 0, 123}, {0, 0, 124}, {0, 0, 126}, {0, 0, 128}, {0, 0, 129}, {0, 0, 130}, {0, 0, 132}, {0, 0, 134}, {0, 0, 135}, {0, 0, 136}, {0, 0, 138}, {0, 0, 140}, {0, 0, 141}, {0, 0, 142}, {0, 0, 144}, {0, 0, 146}, {0, 0, 147}, {0, 0, 148}, {0, 0, 150}, {0, 0, 152}, {0, 0, 153}, {0, 0, 154}, {0, 0, 156}, {0, 0, 158}, {0, 0, 159}, {0, 0, 160}, {0, 0, 162}, {0, 0, 164}, {0, 0, 165}, {0, 0, 166}, {0, 0, 168}, {0, 0, 170}, {0, 0, 171}, {0, 0, 172}, {0, 0, 174}, {0, 0, 176}, {0, 0, 177}, {0, 0, 178}, {0, 0, 180}, {0, 0, 182}, {0, 0, 183}, {0, 0, 184}, {0, 0, 186}, {0, 0, 188}, {0, 0, 189}, {0, 0, 190}, {0, 0, 192}, {0, 0, 194}, {0, 0, 195}, {0, 0, 196}, {0, 0, 198}, {0, 0, 200}, {0, 0, 201}, {0, 0, 202}, {0, 0, 204}, {0, 0, 206}, {0, 0, 207}, {0, 0, 208}, {0, 0, 210}, {0, 0, 212}, {0, 0, 213}, {0, 0, 214}, {0, 0, 216}, {0, 0, 218}, {0, 0, 219}, {0, 0, 220}, {0, 0, 222}, {0, 0, 224}, {0, 0, 225}, {0, 0, 226}, {0, 0, 228}, {0, 0, 230}, {0, 0, 231}, {0, 0, 232}, {0, 0, 234}, {0, 0, 236}, {0, 0, 237}, {0, 0, 238}, {0, 0, 240}, {0, 0, 242}, {0, 0, 243}, {0, 0, 244}, {0, 0, 246}, {0, 0, 248}, {0, 0, 249}, {0, 0, 250}, {0, 0, 252}, {0, 0, 254}, {0, 0, 255}, {3, 3, 255}, {7, 7, 254}, {10, 10, 254}, {14, 14, 253}, {17, 17, 253}, {20, 20, 253}, {24, 24, 252}, {27, 27, 252}, {31, 31, 251}, {34, 34, 251}, {37, 37, 250}, {41, 41, 250}, {44, 44, 250}, {48, 48, 249}, {51, 51, 249}, {54, 54, 248}, {58, 58, 248}, {61, 61, 248}, {65, 65, 247}, {68, 68, 247}, {71, 71, 246}, {75, 75, 246}, {78, 78, 245}, {82, 82, 245}, {85, 85, 245}, {88, 88, 244}, {92, 92, 244}, {95, 95, 243}, {99, 99, 243}, {102, 102, 243}, {105, 105, 242}, {109, 109, 242}, {112, 112, 241}, {116, 116, 241}, {119, 119, 241}, {122, 122, 240}, {126, 126, 240}, {129, 129, 239}, {133, 133, 239}, {136, 136, 238}, {139, 139, 238}, {143, 143, 238}, {146, 146, 237}, {150, 150, 237}, {153, 153, 236}, {156, 156, 236}, {160, 160, 236}, {163, 163, 235}, {167, 167, 235}, {170, 170, 234}, {173, 173, 234}, {177, 177, 234}, {180, 180, 233}, {184, 184, 233}, {187, 187, 232}, {190, 190, 232}, {194, 194, 231}, {197, 197, 231}, {201, 201, 231}, {204, 204, 230}, {207, 207, 230}, {211, 211, 229}, {214, 214, 229}, {218, 218, 229}, {221, 221, 228}, {224, 224, 228}, {228, 228, 227}, {231, 231, 227}, {235, 235, 226}, {238, 238, 226}, {241, 241, 226}, {245, 245, 225}, {248, 248, 225}, {252, 252, 224}, {255, 255, 224}, {255, 255, 227}, {255, 255, 230}, {255, 255, 234}, {255, 255, 237}, {255, 255, 240}, {254, 254, 242}, {253, 253, 244}, {252, 252, 246}, {251, 251, 248}, {250, 250, 250}] ("Array 2") cluster{u8, u8, u8}[] [{0, 0, 0}, {3, 0, 0}, {6, 0, 0}, {9, 0, 0}, {12, 0, 0}, {15, 0, 0}, {18, 0, 0}, {21, 0, 0}, {24, 0, 0}, {27, 0, 0}, {30, 0, 0}, {33, 0, 0}, {36, 0, 0}, {39, 0, 0}, {42, 0, 0}, {45, 0, 0}, {48, 0, 0}, {51, 0, 0}, {54, 0, 0}, {57, 0, 0}, {60, 0, 0}, {63, 0, 0}, {66, 0, 0}, {69, 0, 0}, {72, 0, 0}, {75, 0, 0}, {78, 0, 0}, {81, 0, 0}, {84, 0, 0}, {87, 0, 0}, {90, 0, 0}, {93, 0, 0}, {96, 0, 0}, {99, 0, 0}, {102, 0, 0}, {105, 0, 0}, {108, 0, 0}, {111, 0, 0}, {114, 0, 0}, {117, 0, 0}, {120, 0, 0}, {123, 0, 0}, {126, 0, 0}, {129, 0, 0}, {132, 0, 0}, {135, 0, 0}, {138, 0, 0}, {141, 0, 0}, {144, 0, 0}, {147, 0, 0}, {150, 0, 0}, {153, 0, 0}, {156, 0, 0}, {159, 0, 0}, {162, 0, 0}, {165, 0, 0}, {168, 0, 0}, {171, 0, 0}, {174, 0, 0}, {177, 0, 0}, {180, 0, 0}, {183, 0, 0}, {186, 0, 0}, {189, 0, 0}, {192, 0, 0}, {195, 0, 0}, {198, 0, 0}, {201, 0, 0}, {204, 0, 0}, {207, 0, 0}, {210, 0, 0}, {213, 0, 0}, {216, 0, 0}, {219, 0, 0}, {222, 0, 0}, {225, 0, 0}, {228, 0, 0}, {231, 0, 0}, {234, 0, 0}, {237, 0, 0}, {240, 0, 0}, {243, 0, 0}, {246, 0, 0}, {249, 0, 0}, {252, 0, 0}, {255, 0, 0}, {255, 3, 0}, {255, 6, 0}, {255, 9, 0}, {255, 12, 0}, {255, 15, 0}, {255, 18, 0}, {255, 21, 0}, {255, 24, 0}, {255, 27, 0}, {255, 30, 0}, {255, 33, 0}, {255, 36, 0}, {255, 39, 0}, {255, 42, 0}, {255, 45, 0}, {255, 48, 0}, {255, 51, 0}, {255, 54, 0}, {255, 57, 0}, {255, 60, 0}, {255, 63, 0}, {255, 66, 0}, {255, 69, 0}, {255, 72, 0}, {255, 75, 0}, {255, 78, 0}, {255, 81, 0}, {255, 84, 0}, {255, 87, 0}, {255, 90, 0}, {255, 93, 0}, {255, 96, 0}, {255, 100, 0}, {255, 103, 0}, {255, 106, 0}, {255, 109, 0}, {255, 112, 0}, {255, 115, 0}, {255, 118, 0}, {255, 121, 0}, {255, 124, 0}, {255, 127, 0}, {255, 130, 0}, {255, 132, 0}, {255, 135, 0}, {255, 137, 0}, {255, 140, 0}, {255, 143, 0}, {255, 146, 0}, {255, 149, 0}, {255, 152, 0}, {255, 156, 0}, {255, 159, 0}, {255, 162, 0}, {255, 165, 0}, {255, 168, 0}, {255, 171, 0}, {255, 174, 0}, {255, 177, 0}, {255, 180, 0}, {255, 183, 0}, {255, 186, 0}, {255, 189, 0}, {255, 191, 0}, {255, 194, 0}, {255, 197, 0}, {255, 200, 0}, {255, 203, 0}, {255, 206, 0}, {255, 209, 0}, {255, 212, 0}, {255, 215, 0}, {255, 218, 0}, {255, 221, 0}, {255, 224, 0}, {255, 227, 0}, {255, 230, 0}, {255, 233, 0}, {255, 237, 0}, {255, 240, 0}, {255, 243, 0}, {255, 246, 0}, {255, 249, 0}, {255, 252, 0}, {255, 255, 0}, {255, 255, 3}, {255, 255, 6}, {255, 255, 9}, {255, 255, 12}, {255, 255, 15}, {255, 255, 18}, {255, 255, 21}, {255, 255, 24}, {255, 255, 27}, {255, 255, 30}, {255, 255, 33}, {255, 255, 36}, {255, 255, 39}, {255, 255, 42}, {255, 255, 45}, {255, 255, 48}, {255, 255, 51}, {255, 255, 54}, {255, 255, 57}, {255, 255, 60}, {255, 255, 63}, {255, 255, 66}, {255, 255, 69}, {255, 255, 72}, {255, 255, 75}, {255, 255, 78}, {255, 255, 81}, {255, 255, 84}, {255, 255, 87}, {255, 255, 90}, {255, 255, 93}, {255, 255, 96}, {255, 255, 99}, {255, 255, 102}, {255, 255, 105}, {255, 255, 108}, {255, 255, 111}, {255, 255, 113}, {255, 255, 116}, {255, 255, 119}, {255, 255, 122}, {255, 255, 125}, {255, 255, 128}, {255, 255, 131}, {255, 255, 134}, {255, 255, 137}, {255, 255, 140}, {255, 255, 143}, {255, 255, 146}, {255, 255, 149}, {255, 255, 152}, {255, 255, 155}, {255, 255, 158}, {255, 255, 161}, {255, 255, 164}, {255, 255, 167}, {255, 255, 170}, {255, 255, 173}, {255, 255, 176}, {255, 255, 179}, {255, 255, 182}, {255, 255, 185}, {255, 255, 188}, {255, 255, 191}, {255, 255, 194}, {255, 255, 197}, {255, 255, 200}, {255, 255, 203}, {255, 255, 206}, {255, 255, 209}, {255, 255, 212}, {255, 255, 215}, {255, 255, 218}, {255, 255, 221}, {255, 255, 224}, {255, 255, 227}, {255, 255, 230}, {255, 255, 234}, {255, 255, 237}, {255, 255, 240}, {255, 255, 243}, {255, 255, 246}, {255, 255, 249}, {255, 255, 252}, {255, 255, 255}] ("Array 2") cluster{u8, u8, u8}[] [{0, 0, 0}, {2, 0, 0}, {3, 0, 0}, {5, 0, 0}, {7, 0, 0}, {9, 0, 0}, {11, 0, 0}, {13, 0, 3}, {15, 0, 3}, {17, 0, 3}, {19, 0, 3}, {21, 0, 3}, {23, 0, 3}, {25, 0, 3}, {27, 0, 3}, {27, 0, 7}, {31, 0, 7}, {33, 0, 7}, {35, 0, 7}, {37, 0, 7}, {39, 0, 7}, {41, 0, 7}, {43, 0, 7}, {45, 0, 7}, {47, 0, 11}, {49, 0, 11}, {51, 0, 11}, {53, 0, 11}, {55, 0, 11}, {57, 0, 11}, {59, 0, 11}, {59, 3, 11}, {63, 3, 11}, {65, 3, 11}, {67, 3, 11}, {69, 3, 11}, {71, 3, 15}, {73, 3, 15}, {75, 3, 15}, {79, 3, 15}, {81, 3, 15}, {83, 3, 15}, {85, 3, 15}, {87, 3, 15}, {87, 7, 15}, {91, 7, 15}, {93, 7, 15}, {95, 7, 15}, {97, 7, 15}, {99, 7, 15}, {101, 7, 15}, {103, 7, 15}, {105, 7, 15}, {107, 11, 15}, {109, 11, 15}, {111, 11, 15}, {113, 11, 15}, {115, 11, 15}, {117, 11, 15}, {119, 11, 15}, {123, 11, 15}, {125, 11, 15}, {127, 15, 15}, {129, 15, 15}, {131, 15, 19}, {133, 15, 19}, {135, 15, 19}, {137, 15, 19}, {139, 15, 19}, {139, 19, 19}, {143, 19, 19}, {145, 19, 19}, {147, 19, 19}, {149, 19, 19}, {151, 23, 19}, {153, 23, 19}, {155, 23, 19}, {156, 23, 19}, {157, 23, 19}, {159, 27, 19}, {161, 27, 19}, {163, 27, 19}, {165, 27, 19}, {166, 31, 19}, {167, 31, 19}, {169, 31, 19}, {171, 31, 19}, {171, 35, 19}, {175, 35, 19}, {176, 35, 19}, {177, 35, 19}, {179, 39, 19}, {180, 39, 19}, {181, 39, 19}, {183, 43, 19}, {185, 43, 19}, {187, 43, 19}, {187, 47, 19}, {189, 47, 19}, {191, 47, 19}, {191, 51, 19}, {192, 51, 19}, {191, 51, 19}, {195, 55, 19}, {195, 57, 19}, {195, 59, 19}, {199, 59, 19}, {199, 61, 19}, {199, 63, 19}, {201, 63, 19}, {203, 67, 19}, {204, 67, 19}, {205, 69, 19}, {207, 71, 19}, {207, 73, 19}, {207, 75, 19}, {207, 77, 19}, {209, 79, 19}, {211, 79, 19}, {211, 83, 19}, {211, 85, 19}, {211, 87, 19}, {213, 87, 19}, {215, 91, 19}, {215, 93, 19}, {215, 95, 19}, {215, 97, 19}, {217, 99, 19}, {219, 99, 19}, {219, 103, 19}, {219, 105, 19}, {219, 106, 19}, {219, 107, 19}, {219, 111, 19}, {221, 111, 19}, {223, 115, 19}, {223, 117, 23}, {223, 119, 23}, {223, 121, 23}, {223, 123, 23}, {223, 125, 23}, {225, 127, 23}, {227, 127, 23}, {227, 131, 23}, {227, 133, 27}, {227, 135, 27}, {227, 137, 27}, {227, 139, 27}, {227, 141, 29}, {229, 143, 31}, {231, 143, 31}, {231, 145, 31}, {231, 147, 31}, {231, 149, 31}, {231, 151, 35}, {231, 153, 35}, {231, 155, 35}, {233, 157, 35}, {235, 159, 37}, {235, 160, 39}, {235, 161, 39}, {235, 163, 39}, {235, 165, 43}, {235, 167, 43}, {235, 169, 45}, {235, 171, 47}, {235, 171, 47}, {237, 173, 47}, {239, 175, 49}, {239, 177, 51}, {239, 179, 51}, {239, 179, 53}, {239, 179, 55}, {239, 183, 59}, {239, 185, 59}, {239, 187, 61}, {239, 187, 63}, {239, 189, 65}, {241, 191, 67}, {243, 191, 69}, {243, 191, 71}, {243, 191, 73}, {243, 191, 75}, {243, 197, 75}, {243, 199, 79}, {243, 201, 81}, {243, 203, 83}, {243, 203, 85}, {243, 205, 87}, {243, 207, 87}, {243, 207, 91}, {245, 209, 93}, {247, 211, 95}, {247, 211, 97}, {247, 213, 99}, {247, 215, 103}, {247, 215, 105}, {247, 215, 107}, {247, 219, 107}, {247, 219, 111}, {247, 221, 113}, {247, 223, 115}, {247, 223, 119}, {247, 223, 121}, {247, 223, 123}, {247, 227, 123}, {247, 227, 127}, {247, 227, 129}, {247, 229, 131}, {247, 231, 135}, {249, 231, 135}, {251, 231, 139}, {251, 231, 143}, {251, 235, 143}, {251, 235, 147}, {251, 235, 149}, {251, 235, 151}, {251, 237, 153}, {251, 239, 155}, {251, 239, 159}, {251, 239, 161}, {251, 239, 163}, {251, 241, 167}, {251, 243, 167}, {251, 243, 171}, {251, 243, 173}, {251, 243, 175}, {251, 243, 179}, {251, 245, 181}, {251, 247, 183}, {251, 247, 187}, {251, 247, 189}, {251, 247, 191}, {251, 247, 193}, {251, 247, 195}, {251, 247, 199}, {251, 249, 201}, {251, 251, 203}, {251, 251, 207}, {251, 251, 209}, {251, 251, 211}, {251, 251, 213}, {251, 251, 215}, {251, 251, 219}, {251, 251, 221}, {251, 251, 223}, {251, 251, 227}, {251, 251, 229}, {251, 251, 231}, {251, 251, 235}, {251, 251, 237}, {251, 251, 239}, {251, 251, 243}, {251, 251, 245}, {251, 251, 247}, {251, 251, 251}] ("Array")] -> w236
              frame "Gray", Default {
              }
              frame "Red" {
              }
              frame "Green" {
              }
              frame "Blue" {
              }
              frame "Cyan" {
              }
              frame "Magenta" {
              }
              frame "Yellow" {
              }
              frame "Red-White" {
              }
              frame "Green-White" {
              }
              frame "Blue-White" {
              }
              frame "Fire" {
              }
              frame "Glow" {
              }
            }
            n130 = To More Specific Class(target class=w241, reference=w240) -> (specific class reference=w239:refnum<vi>)  [unwired: 1 in, 1 out]
            n131 = property class="ImageControl"(reference=w239, "Palette Type"=w237) -> (reference out=w238:refnum<vi>)  [unwired: 1 in, 1 out]
            n132 = property class="ImageControl"(reference=w249, "User Palette"=w236) -> ()  [unwired: 1 in, 2 out]
            n133 = property class="ImageControl"(reference=w238, "User Palette"=w236) -> ()  [unwired: 1 in, 2 out]
          }
          frame "Line Tool", "Pan Tool", "Point Tool", "Rectangle Tool", "Zoom Tool" {
            w270 = u32 0 items=["Zoom Tool"=8, "Selection Tool"=0, "Pan Tool"=9, "Point Tool"=1, "Line Tool"=2, "Rectangle Tool"=3, "Rotated Rectangle Tool"=12, "Polyline Tool"=10, "Polygon Tool"=5, "Freehand Tool"=11, "Closed Freehand Tool"=6, "Ellipse Tool"=4, "Annulus Tool"=7] ("Current ROI Tool")
            n134 = case shown="Default" w267 {
              tunnel: [w274 w275 w276 w277 w278 w279] -> w266
              frame Default {
                w274 = u32 0 items=["Zoom Tool"=8, "Selection Tool"=0, "Pan Tool"=9, "Point Tool"=1, "Line Tool"=2, "Rectangle Tool"=3, "Rotated Rectangle Tool"=12, "Polyline Tool"=10, "Polygon Tool"=5, "Freehand Tool"=11, "Closed Freehand Tool"=6, "Ellipse Tool"=4, "Annulus Tool"=7] ("Current ROI Tool")
              }
              frame "Line Tool" {
                w275 = u32 2 items=["Zoom Tool"=8, "Selection Tool"=0, "Pan Tool"=9, "Point Tool"=1, "Line Tool"=2, "Rectangle Tool"=3, "Rotated Rectangle Tool"=12, "Polyline Tool"=10, "Polygon Tool"=5, "Freehand Tool"=11, "Closed Freehand Tool"=6, "Ellipse Tool"=4, "Annulus Tool"=7] ("Current ROI Tool")
              }
              frame "Pan Tool" {
                w276 = u32 9 items=["Zoom Tool"=8, "Selection Tool"=0, "Pan Tool"=9, "Point Tool"=1, "Line Tool"=2, "Rectangle Tool"=3, "Rotated Rectangle Tool"=12, "Polyline Tool"=10, "Polygon Tool"=5, "Freehand Tool"=11, "Closed Freehand Tool"=6, "Ellipse Tool"=4, "Annulus Tool"=7] ("Current ROI Tool")
              }
              frame "Point Tool" {
                w277 = u32 1 items=["Zoom Tool"=8, "Selection Tool"=0, "Pan Tool"=9, "Point Tool"=1, "Line Tool"=2, "Rectangle Tool"=3, "Rotated Rectangle Tool"=12, "Polyline Tool"=10, "Polygon Tool"=5, "Freehand Tool"=11, "Closed Freehand Tool"=6, "Ellipse Tool"=4, "Annulus Tool"=7] ("Current ROI Tool")
              }
              frame "Rectangle Tool" {
                w278 = u32 3 items=["Zoom Tool"=8, "Selection Tool"=0, "Pan Tool"=9, "Point Tool"=1, "Line Tool"=2, "Rectangle Tool"=3, "Rotated Rectangle Tool"=12, "Polyline Tool"=10, "Polygon Tool"=5, "Freehand Tool"=11, "Closed Freehand Tool"=6, "Ellipse Tool"=4, "Annulus Tool"=7] ("Current ROI Tool")
              }
              frame "Zoom Tool" {
                w279 = u32 8 items=["Zoom Tool"=8, "Selection Tool"=0, "Pan Tool"=9, "Point Tool"=1, "Line Tool"=2, "Rectangle Tool"=3, "Rotated Rectangle Tool"=12, "Polyline Tool"=10, "Polygon Tool"=5, "Freehand Tool"=11, "Closed Freehand Tool"=6, "Ellipse Tool"=4, "Annulus Tool"=7] ("Current ROI Tool")
              }
            }
            n135 = property class="ImageControl"(reference=w273) -> (reference out=w269:refnum<vi>, "Current ROI Tool"=w272:u32)  [unwired: 1 in, 1 out]
            n136 = Equal?(x=w272, y=w266) -> (x = y?=w271:bool)
            n137 = Select(t=w270, s=w271, f=w266) -> (s? t:f=w268:u32)
            n138 = property class="ImageControl"(reference=w269, "Current ROI Tool"=w268) -> ()  [unwired: 1 in, 2 out]
          }
          frame "Auto Scale Z" {
            w304 = u32 14 items=["Default"=10, "Most Significant Bits"=11, "Full Dynamic"=12, "Downshift"=13, "Given Range"=14, "90% Dynamic"=15, "Given Percent Range"=16] ("16-bit Display Mapping:Conversion Method")
            w303 = u32 10 items=["Default"=10, "Most Significant Bits"=11, "Full Dynamic"=12, "Downshift"=13, "Given Range"=14, "90% Dynamic"=15, "Given Percent Range"=16] ("16-bit Display Mapping:Conversion Method")
            n139 = for {
              tunnel: w301 -> [w309] mode=indexing
              tunnel: w298 -> [w310]
              tunnel: [w308] -> w299
              i -> [w308]
              stop <- w311 stop-if-true
              n140 = Equal?(x=w310, y=w309) -> (x = y?=w311:bool)
            }
            n141 = property class="ImageControl"(reference=w298) -> (reference out=w307:refnum<vi>, "16-bit Display Conversion Method"=w306:u32, "Value"=w288:variant)  [unwired: 1 in, 1 out]
            n142 = Index Array(array=w300, index=w299) -> (element=w297:refnum<vi>)
            n143 = property class="Clust (strict)"(reference=w297) -> ("Controls[]"=w296:refnum<vi>[])  [unwired: 1 in, 2 out]
            n144 = Variant To Data(type=T2 refnum ("New Image"), Variant=w288) -> (data=w286:T2)  [unwired: 1 in, 1 out]
            n145 = call "IMAQ Quantify 2"("Image"=w286) -> ("Global Report"=w287:T14)  [unwired: 8 in, 2 out]
            n146 = Equal?(x=w306, y=w303) -> (x = y?=w305:bool)
            n147 = Unbundle By Name(w287) -> ("Maximal Value"=w283:sgl, "Minimal Value"=w282:sgl)
            n148 = Select(t=w304, s=w305, f=w303) -> (s? t:f=w302:u32)
            n149 = To Long Integer(number=w283) -> (32bit integer=w285:i32)
            n150 = To Long Integer(number=w282) -> (32bit integer=w284:i32)
            n151 = To Single Precision Float(number=w283) -> (single precision float=w280:sgl)
            n152 = To Single Precision Float(number=w282) -> (single precision float=w281:sgl)
            n153 = property class="ImageControl"(reference=w307, "16-bit Display Conversion Method"=w302, "16-bit Display Maximum Value"=w285, "16-bit Display Minimum Value"=w284) -> ()  [unwired: 1 in, 2 out]
            n154 = Index Array(array=w296, index #1=2 ("index"), index #2=1 ("index")) -> (element #1=w293:refnum<vi>, element #2=w290:refnum<vi>)
            n155 = To Variant(anything=w280) -> (Variant=w292:variant)
            n156 = To Variant(anything=w281) -> (Variant=w291:variant)
            n157 = property class="Ctl"(reference=w293, "Value"=w292) -> ()  [unwired: 1 in, 2 out]
            n158 = property class="Ctl"(reference=w290, "Value"=w291) -> ()  [unwired: 1 in, 2 out]
          }
          frame "Auto Scale All" {
            n159 = for {
              tunnel: w312 -> [w314] mode=indexing
              w313 = u32 10 items=["Default"=10, "Most Significant Bits"=11, "Full Dynamic"=12, "Downshift"=13, "Given Range"=14, "90% Dynamic"=15, "Given Percent Range"=16] ("16-bit Display Mapping:Conversion Method")
              n160 = property class="ImageControl"(reference=w314, "16-bit Display Conversion Method"=w313) -> ()  [unwired: 1 in, 2 out]
            }
          }
          frame "Show Z Scale" {
            n161 = for {
              tunnel: w322 -> [w326] mode=indexing
              tunnel: w320 -> [w324]
              tunnel: [w323] -> w319
              i -> [w323]
              stop <- w325 stop-if-true
              n162 = Equal?(x=w324, y=w326) -> (x = y?=w325:bool)
            }
            n163 = Index Array(array=w321, index=w319) -> (element=w318:refnum<vi>)
            n164 = property class="Clust (strict)"(reference=w318) -> (reference out=w317:refnum<vi>, "Visible"=w316:bool)  [unwired: 1 in, 1 out]
            n165 = Not(x=w316) -> (.not. x?=w315:bool)
            n166 = property class="Clust (strict)"(reference=w317, "Visible"=w315) -> ()  [unwired: 1 in, 2 out]
          }
          frame "Lock All AutoScale" {
            n167 = call "Lock Displays AE.vi"("Action"=Display_Module_Standard_Action."Read") -> ("Lock All Markers Out"=w332:bool, "Lock All AutoScale Out"=w330:bool, "Lock Pan/Zoom Out"=w329:bool)  [unwired: 12 in]
            n168 = Not(x=w330) -> (.not. x?=w331:bool)
            n169 = call "Lock Displays AE.vi"("Lock All Markers"=w332, "Action"=Display_Module_Standard_Action."Write", "Lock All AutoScale"=w331, "Lock Pan/Zoom"=w329) -> ()  [unwired: 9 in, 3 out]
          }
          frame "Lock All Markers" {
            n170 = property class="ImageControl"(reference=w334) -> ("ROI"=w335:T11)  [unwired: 1 in, 2 out]
            n171 = call "Lock Displays AE.vi"("Action"=Display_Module_Standard_Action."Read") -> ("Lock All Markers Out"=w339:bool, "Lock All AutoScale Out"=w336:bool, "Lock Pan/Zoom Out"=w341:bool)  [unwired: 12 in]
            n172 = Not(x=w339) -> (.not. x?=w340:bool)
            n173 = call "Lock Displays AE.vi"("Lock All Markers"=w340, "Action"=Display_Module_Standard_Action."Write", "Lock All AutoScale"=w336, "Lock Pan/Zoom"=w341) -> ()  [unwired: 9 in, 3 out]
            n174 = for {
              tunnel: w333 -> [w343] mode=indexing
              tunnel: w335 -> [w342]
              n175 = property class="ImageControl"(reference=w343, "ROI"=w342) -> ()  [unwired: 1 in, 2 out]
            }
          }
          frame "Lock Zoom/Pan" {
            n176 = property class="ImageControl"(reference=w344) -> ("ZoomSingle"=w347:cluster{"X":sgl, "Y":sgl}, "Image Center Position"=w346:cluster{"X":u32, "Y":u32})  [unwired: 1 in, 2 out]
            n177 = call "Lock Displays AE.vi"("Action"=Display_Module_Standard_Action."Read") -> ("Lock All Markers Out"=w351:bool, "Lock All AutoScale Out"=w350:bool, "Lock Pan/Zoom Out"=w348:bool)  [unwired: 12 in]
            n178 = Not(x=w348) -> (.not. x?=w349:bool)
            n179 = call "Lock Displays AE.vi"("Lock All Markers"=w351, "Action"=Display_Module_Standard_Action."Write", "Lock All AutoScale"=w350, "Lock Pan/Zoom"=w349) -> ()  [unwired: 9 in, 3 out]
            n180 = for {
              tunnel: w345 -> [w356] mode=indexing
              tunnel: w347 -> [w355]
              tunnel: w346 -> [w354]
              n181 = property class="ImageControl"(reference=w356, "ZoomSingle"=w355, "Image Center Position"=w354) -> ()  [unwired: 1 in, 2 out]
            }
          }
          frame "Clear All Markers", "Clear Markers" {
            n182 = Build Array(w361) -> (w360:refnum<vi>[])
            n183 = Equal?(x="Clear Markers", y=w363) -> (x = y?=w358:bool)
            n184 = Select(t=w360, s=w358, f=w359) -> (s? t:f=w357:refnum<vi>[])
            n185 = for {
              tunnel: w357 -> [w364] mode=indexing
              n186 = property class="ImageControl"(reference=w364, "ROI"=T11 {"Global Rectangle"=[], "Contours"=[]}) -> ("Value"=w365:variant)  [unwired: 1 in, 2 out]
              n187 = Variant To Data(type=T2 refnum ("New Image"), Variant=w365) -> (data=w368:T2)  [unwired: 1 in, 1 out]
              n188 = Not A Number/Path/Refnum?(number/path/refnum=w368) -> (NaN/Path/Refnum?=w367:bool)
              n189 = case shown="False" w367 {
                tunnel: w368 -> [w376 _]
                frame False {
                  w370 = "Image ROI" ("element")
                  n190 = call "IMAQ Clear Overlay"("Image"=w376) -> ("Image Out"=w375:T2)  [unwired: 9 in, 1 out]
                  n191 = call "IMAQ Get Custom Keys"("Image"=w375) -> ("Keys"=w374:string[], "Image (duplicate)"=w371:T2)  [unwired: 7 in, 2 out]
                  n192 = Search 1D Array(1D array=w374, element=w370) -> (index of element=w373:i32)  [unwired: 1 in]
                  n193 = Less Than 0?(x=w373) -> (x < 0?=w372:bool)
                  n194 = case shown="False" w372 {
                    tunnel: w371 -> [w378 _]
                    tunnel: w370 -> [w377 _]
                    frame False {
                      n195 = call "IMAQ Remove Custom Data"("Key"=w377, "Image"=w378) -> ()  [unwired: 7 in, 3 out]
                    }
                    frame True {
                    }
                  }
                }
                frame True {
                }
              }
            }
          }
          frame "Reset Zoom" {
            n196 = call "Lock Displays AE.vi"("Action"=Display_Module_Standard_Action."Read") -> ("Lock Pan/Zoom Out"=w383:bool)  [unwired: 12 in, 2 out]
            n197 = Build Array(w385) -> (w380:refnum<vi>[])
            n198 = Not(x=w383) -> (.not. x?=w382:bool)
            n199 = Select(t=w380, s=w382, f=w381) -> (s? t:f=w379:refnum<vi>[])
            n200 = for {
              tunnel: w379 -> [w389] mode=indexing
              w386 = u32 0 items=["Zoom Tool"=8, "Selection Tool"=0, "Pan Tool"=9, "Point Tool"=1, "Line Tool"=2, "Rectangle Tool"=3, "Rotated Rectangle Tool"=12, "Polyline Tool"=10, "Polygon Tool"=5, "Freehand Tool"=11, "Closed Freehand Tool"=6, "Ellipse Tool"=4, "Annulus Tool"=7] ("Current ROI Tool")
              n201 = property class="ImageControl"(reference=w389, "Zoom to Fit Mode"=TRUE) -> (reference out=w387:refnum<vi>)  [unwired: 1 in, 1 out]
              n202 = property class="ImageControl"(reference=w387, "Current ROI Tool"=w386) -> ()  [unwired: 1 in, 2 out]
            }
          }
          frame "Load Image" {
          }
        }
      }
      event "Channel 1", "Channel 2", "Channel 3", "Channel 4", "Channel 5", "Channel 6": Mouse Up {
        # "1: Left Click\n2: Right Click\n3: Middle Click"
        n203 = event-data() -> ("CtlRef"=w391:refnum<vi>)  [unwired: 1 in, 1 out]
        n204 = property class="ImageControl"(reference=w391) -> ("ZoomSingle"=w399:cluster{"X":sgl, "Y":sgl}, "Image Center Position"=w395:cluster{"X":u32, "Y":u32})  [unwired: 1 in, 2 out]
        n205 = property class="ImageControl" props=["ROI", "Value"](reference=w391) -> ("ROI"=w392:T11)  [unwired: 1 in, 3 out]
        n206 = call "Lock Displays AE.vi"("Action"=Display_Module_Standard_Action."Read") -> ("Lock Pan/Zoom Out"=w396:bool)  [unwired: 12 in, 2 out]
        n207 = call "Lock Displays AE.vi"("Action"=Display_Module_Standard_Action."Read") -> ("Lock All Markers Out"=w400:bool)  [unwired: 12 in, 2 out]
        n208 = case shown="True" w396 {
          tunnel: w397 -> [_ w412]
          tunnel: w399 -> [_ w411]
          tunnel: w395 -> [_ w410]
          frame False {
          }
          frame True {
            n209 = for {
              tunnel: w412 -> [w415] mode=indexing
              tunnel: w411 -> [w414]
              tunnel: w410 -> [w413]
              n210 = property class="ImageControl"(reference=w415, "ZoomSingle"=w414, "Image Center Position"=w413) -> ()  [unwired: 1 in, 2 out]
            }
          }
        }
        n211 = case shown="True" w400 {
          tunnel: w397 -> [_ w417]
          tunnel: w392 -> [_ w416]
          frame False {
          }
          frame True {
            n212 = for {
              tunnel: w417 -> [w419] mode=indexing
              tunnel: w416 -> [w418]
              n213 = property class="ImageControl"(reference=w419, "ROI"=w418) -> ()  [unwired: 1 in, 2 out]
            }
          }
        }
        n214 = Unbundle By Name(w392) -> ("Contours"=w394:T15)
        n215 = Array Size(array=w394) -> (size(s)=w390:i32)
        n216 = Equal To 0?(x=w390) -> (x = 0?=w393:bool)
        n217 = case shown="False" w393 {
          tunnel: w392 -> [w409 _]
          tunnel: w391 -> [w408 _]
          frame False {
            n218 = property class="ImageControl"(reference=w408) -> ("Value"=w405:variant)  [unwired: 1 in, 2 out]
            n219 = Flatten To JSON(anything=w409) -> (JSON string=w406:string)  [unwired: 2 in, 1 out]
            n220 = Variant To Data(type=T2 refnum ("New Image"), Variant=w405) -> (data=w403:T2)  [unwired: 1 in, 1 out]
            n221 = call "IMAQ Write Custom Data"("Custom Data In"=w406, "Key"="Image ROI", "Image"=w403) -> ()  [unwired: 7 in, 2 out]
          }
          frame True {
          }
        }
      }
      event "Channel 1", "Channel 2", "Channel 3", "Channel 4", "Channel 6", "Channel 5": Mouse Enter; "Channel 1", "Channel 2", "Channel 3", "Channel 4", "Channel 5", "Channel 6": Mouse Leave {
        w420 = Display_Module_Standard_Action."Write" ("Action")
        n222 = event-data() -> ("Type"=w423:T10, "CtlRef"=w422:refnum<vi>)  [unwired: 1 in]
        n223 = call "Current Display Mouse.vi"("Event Type"=w423, "Action"=w420, "IMAQ Image Display Ref"=w422) -> ()  [unwired: 11 in, 2 out]
        n224 = call "Main Info Bar Message AE.vi"("Action"=w420, "Message"="") -> ()  [unwired: 13 in, 1 out]
      }
      event Value Change {
        w430 = u32 14 items=["Default"=10, "Most Significant Bits"=11, "Full Dynamic"=12, "Downshift"=13, "Given Range"=14, "90% Dynamic"=15, "Given Percent Range"=16] ("16-bit Display Mapping:Conversion Method")
        n225 = event-data() -> ("OldVal.Z Scale Max"=w427:sgl, "OldVal.Z Scale Min"=w428:sgl, "CtlRef"=w429:refnum<vi>)  [unwired: 1 in]
        n226 = for {
          tunnel: w434 -> [w436] mode=indexing
          tunnel: [w438] -> w432
          tunnel: w429 -> [w437]
          i -> [w438]
          stop <- w439 stop-if-true
          n227 = Equal?(x=w437, y=w436) -> (x = y?=w439:bool)
        }
        n228 = To Long Integer(number=w427) -> (32bit integer=w426:i32)
        n229 = To Long Integer(number=w428) -> (32bit integer=w425:i32)
        n230 = Index Array(array=w433, index=w432) -> (element=w431:refnum<vi>)
        n231 = property class="ImageControl"(reference=w431, "16-bit Display Maximum Value"=w426, "16-bit Display Minimum Value"=w425, "16-bit Display Conversion Method"=w430) -> ()  [unwired: 1 in, 2 out]
      }
      event Key Down; Key Up {
        # "Switch to the Pan Tool when the space bar is held down"
        n232 = event-data() -> ("Type"=w446:T10, "ScanCode"=w444:i16)  [unwired: 1 in]
        n233 = Equal?(x=lveventtype."Key Down", y=w446) -> (x = y?=w440:bool)
        n234 = Equal?(x=w444, y=i16 57) -> (x = y?=w442:bool)
        n235 = case shown="True" w442 {
          tunnel: w441 -> [_ w452]
          tunnel: w440 -> [_ w451]
          frame False {
          }
          frame True {
            w449 = u32 0 items=["Zoom Tool"=8, "Selection Tool"=0, "Pan Tool"=9, "Point Tool"=1, "Line Tool"=2, "Rectangle Tool"=3, "Rotated Rectangle Tool"=12, "Polyline Tool"=10, "Polygon Tool"=5, "Freehand Tool"=11, "Closed Freehand Tool"=6, "Ellipse Tool"=4, "Annulus Tool"=7] ("Current ROI Tool")
            w450 = u32 9 items=["Zoom Tool"=8, "Selection Tool"=0, "Pan Tool"=9, "Point Tool"=1, "Line Tool"=2, "Rectangle Tool"=3, "Rotated Rectangle Tool"=12, "Polyline Tool"=10, "Polygon Tool"=5, "Freehand Tool"=11, "Closed Freehand Tool"=6, "Ellipse Tool"=4, "Annulus Tool"=7] ("Current ROI Tool")
            n236 = Select(t=w450, s=w451, f=w449) -> (s? t:f=w448:u32)
            n237 = for {
              tunnel: w452 -> [w454] mode=indexing
              tunnel: w448 -> [w453]
              n238 = property class="ImageControl"(reference=w454, "Current ROI Tool"=w453) -> ()  [unwired: 1 in, 2 out]
            }
          }
        }
      }
      event "Exit": Value Change {
        n239 = event-data() -> ("NewVal"=w459:bool)  [unwired: 1 in]
        n240 = Close Reference(reference=w458) -> ()  [unwired: 1 in, 1 out]
        n241 = call "IMAQ Dispose"("Image"=w457) -> ()  [unwired: 5 in, 1 out]
        n242 = call "Main Info Bar Message AE.vi"("Action"=Display_Module_Standard_Action."Write", "Message"="") -> ()  [unwired: 13 in, 1 out]
      }
    }
  }
  n243 = Initialize Array(T2 refnum ("New Image"), 0 ("dimension size")) -> (w30:T2[])
  n244 = property on="Exit" class="Bool (strict)"("Value"=FALSE ("Exit")) -> (error out=w1:errorcluster)  [unwired: 2 in, 1 out]
  n245 = Obtain Notifier(name (unnamed)="Display Module IMAQ Refs", notification data type=w30, create if not found? (T)=TRUE, error in (no error)=w1) -> (notifier out=w4:refnum<notifier>)  [unwired: 2 out]
  n246 = while {
    tunnel: w4 -> [w469]
    tunnel: w29 -> [w465]
    tunnel: [w462] -> w28
    tunnel: w5 -> [w461]
    stop <- "Exit" stop-if-true
    n247 = Get Notifier Status(notifier=w469) -> (notifier out=w462:refnum<notifier>, current notification=w466:T2[])  [unwired: 1 in, 3 out]
    n248 = Array Size(array=w466) -> (size(s)=w460:i32)
    n249 = feedback-in #2(w460) -> ()
    n250 = feedback #2(50) -> (w467:i32)
    n251 = Not Equal?(x=w460, y=w467) -> (x != y?=w463:bool)
    n252 = case shown="False" w463 {
      tunnel: w460 -> [_ w480]
      tunnel: w466 -> [w472 _]
      tunnel: w465 -> [w471 w477]
      tunnel: w461 -> [_ w478]
      frame False {
        # "Normal display mode"
        n253 = for {
          tunnel: w471 -> [w475] mode=indexing
          tunnel: w472 -> [w473] mode=indexing
          n254 = To Variant(anything=w473) -> (Variant=w474:variant)
          n255 = property class="ImageControl"(reference=w475, "Value"=w474) -> ()  [unwired: 1 in, 2 out]
        }
        n256 = Wait (ms)(milliseconds to wait=u32 50) -> ()  [unwired: 1 out]
      }
      frame True {
        # "No. of Refs Changed"
        n257 = To Unsigned Byte Integer(number=w480) -> (unsigned 8bit integer=w481:u8)
        n258 = call "Arrange Displays.vi"("Number of Displays"=w481, "Action"=T8."Change Number", "IMAQ Display Refs"=w477, "Aspect Ratio (Width/Height)"=1.0, "Z Scale Refs"=w478) -> ()  [unwired: 9 in, 2 out]
      }
    }
  }
  n259 = Release Notifier(notifier=w28) -> ()  [unwired: 2 in, 3 out]
